vi "Alicat Full Driver Example.vi"() -> ()   [LabVIEW 2015]
doc: "Example program displaying the potential usage of nearly all of the VI's included in the Alicat LabVIEW Driver Library.\n\nThis VI only connects to a single Alicat at a time, and some features may be locked out due to circuit board revision or firmware revision (newer units have additional features available to them).\n\nIf you have any questions regarding the VI's used in this example, please see the Alicat LabVIEW Driver Library Manual (available on the Alicat website and included in the driver library. If you have remaining questions, please contact Alicat at (520) 290-6060 or info@alicat.com."
panel:
  in  "Tare AP Sensor":bool
  in  "Wait message":cluster{"Boolean":bool}
  in  "Read/Write Options":T1 {"Controller Select" items=["No controller"=0, "Volumetric Flow"=36, "Mass Flow"=37, "Absolute Pressure"=34, "Gauge Pressure"=38, "Differential Pressure"=39]}
  out "Batch Units":string="SL"
  in  "Serial Only":T2={"Valve Drive"=FALSE, "Totalizer"=TRUE, "Totalizer Timer"=FALSE, "Totalizer Peak Flow"=FALSE, "Show Abs., Gauge\nand Baro. pressures"=FALSE}
  in  "Data Logging Options":T3={"Absolute Press."=TRUE, "Gauge/Diff. Press."=TRUE, "Barometric Press."=TRUE, "Temperature"=TRUE, "Volumetric"=TRUE, "Mass Flow"=TRUE, "Setpoint"=TRUE, "Valve Drive"=FALSE, "Totalizer"=TRUE, "Tot. Timer [s]"=FALSE, "Tot. Avg. Flow"=FALSE, "Tot. Peak Flow"=FALSE, "Gas Selected"=TRUE, "Log Data"=FALSE}
  out "Measurement Data":T4
  in  "Chart: Manual Scale Adjust":bool
  in  "Chart: AutoScale":bool=TRUE
  out "Chart":T5(graph)
  out "Register value":string
  in  "Reg. to read":u16
  in  "Read Register":bool
  in  "COMPOSER gas mix input":T6={"Mix % 1"=0.0, "Include # 1"=FALSE, "Mix % 2"=0.0, "Include # 2"=FALSE, "Mix % 3"=0.0, "Include # 3"=FALSE, "Mix % 4"=0.0, "Include # 4"=FALSE, "Mix % 5"=0.0, "Include # 5"=FALSE, "COMPOSER gas 1"=0, "COMPOSER gas 2"=0, "COMPOSER gas 3"=0, "COMPOSER gas 4"=0, "COMPOSER gas 5"=0, "Create COMPOSER Mix"=FALSE, "Mix #"=236, "Mix name"="MyMix1", "Completion\ntext"="", "Create COMPOSER Mix 2"=FALSE} {"Mix #" min=236 max=255 step=1; "COMPOSER gas 5" items=["MyMix1"=236]; "COMPOSER gas 4" items=["MyMix1"=236]; "COMPOSER gas 3" items=["MyMix1"=236]; "COMPOSER gas 2" items=["MyMix1"=236]; "COMPOSER gas 1" items=["MyMix1"=236]; "Mix % 1" min=0.0 max=100.0 step=0.01; "Mix % 2" min=0.0 max=100.0 step=0.01; "Mix % 3" min=0.0 max=100.0 step=0.01; "Mix % 4" min=0.0 max=100.0 step=0.01; "Mix % 5" min=0.0 max=100.0 step=0.01}
  in  "Chart: Setpoint":bool=TRUE
  in  "PID Settings":T7 {"P Gain" min=0 max=65535 step=1; "D Gain" min=0 max=65535 step=1; "I Gain" min=0 max=65535 step=1}
  in  "Log Register Values":bool
  out "Meas. per\nsecond [Hz]":dbl caption="Elapsed Time (s)"
  out "Time between\nreadings [ms]":dbl caption="Elapsed Time (s)"
  in  "Chart: Graphing":bool=TRUE
  out "Read-Only Options":T8={"Analog SP"=enum."4-20mA", "Control Invert"=enum."Pressure", "Main PWM"=enum."Volumetric Flow 0-2.5-5V bidir", "Aux PWM"=enum."Fixed 0.00V"}
  in  "Tare Options":T9={"Display"=enum."None", "External"=enum."None", "Auto-Tare Delay [s]"=nan} {"Auto-Tare Delay [s]" min=0.0 max=25.5 step=0.1 format="%.1g"}
  in  "Tare Pressure":bool
  in  "Tare Flow":bool
  in  "Reset Total":bool
  in  "Chart: Mass Flow":bool=TRUE
  in  "Chart: Volumetric":bool=TRUE
  in  "Chart: Temperature":bool=TRUE
  in  "Chart: Pressure":bool=TRUE
  in  "Time between \nreadings [ms]":u32
  out "Totalizer":T10(ring)
  out "Setpoint Units":string="SLPM"
  in  "Serial and Display":T11={"Pressure"=TRUE, "Temperature"=TRUE, "Volumetric"=TRUE, "Mass Flow"=TRUE, "Tot. Avg Flow"=FALSE, "Gas Selected"=TRUE}
  out "(Full Scale)":dbl=nan
  in  "Setpoint":dbl
  in  "Batch Setpoint":dbl format="%.2f"
  in  "Gas Select":u16(ring) items=["MyMix1"=236]
  out "Manufacturer Info":string
  in  "COM Port Settings":T12={"Unit ID"="A", "Baud Rate"=enum."19200", "VISA Sesssion In"="COM1"}
  # "Setpoint and Batching Controls"
  # "Manual Tare"
  # "Data Frame Enables"
  # "Controller Options\nand Analog Signal\nInformation"
  # "(Resetting the Totalizer will reset the batch)"
  # "Graphing Options:"
  # "VI Timing Options"
  # "Register Values"
  # "Populating VI with device information, please wait."
  # "Altering log options will start a new data log"
  # "(The data will be logged to the folder containing the VI)"
  # "Totalizer Timer"
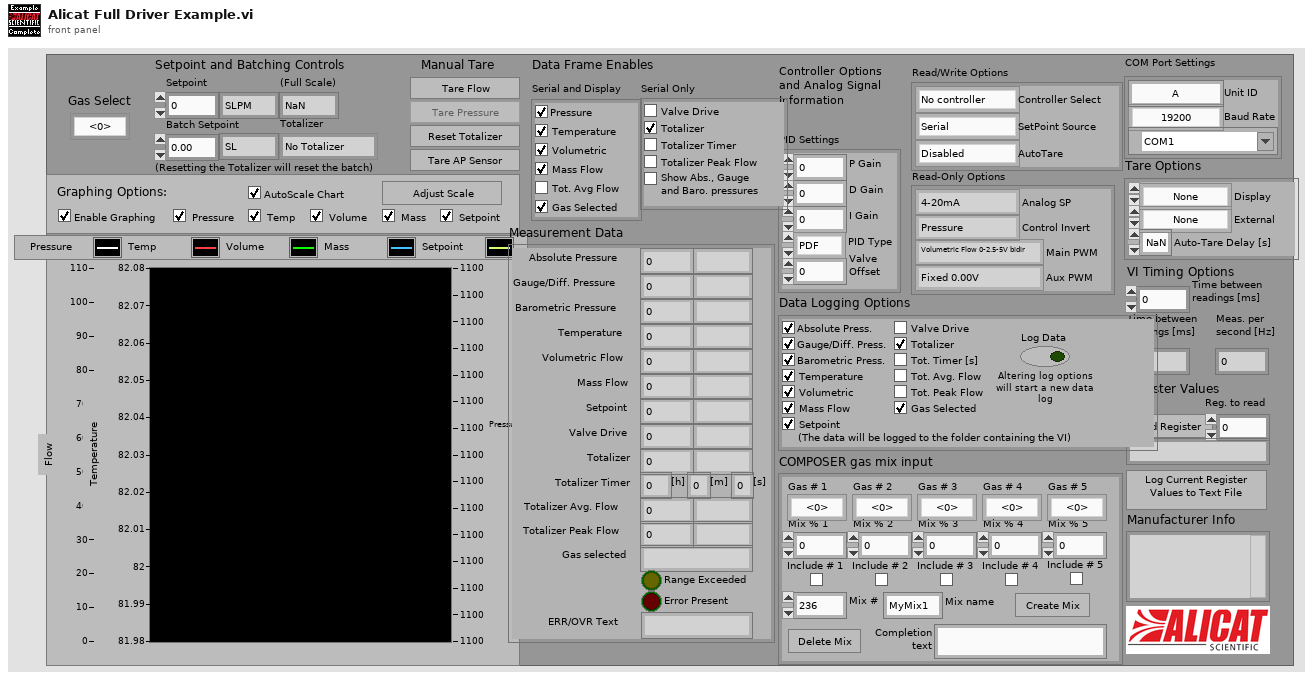
[diagram p1: front panel]
types:
  T1 = cluster{"Controller Select":u16, "SetPoint Source":enum8{"Serial", "Local", "Analog", "Unknown"}, "AutoTare":enum16{"Disabled", "Enabled"}}
  T2 = cluster{"Valve Drive":bool, "Totalizer":bool, "Totalizer Timer":bool, "Totalizer Peak Flow":bool, "Show Abs., Gauge\nand Baro. pressures":bool}
  T3 = cluster{"Absolute Press.":bool, "Gauge/Diff. Press.":bool, "Barometric Press.":bool, "Temperature":bool, "Volumetric":bool, "Mass Flow":bool, "Setpoint":bool, "Valve Drive":bool, "Totalizer":bool, "Tot. Timer [s]":bool, "Tot. Avg. Flow":bool, "Tot. Peak Flow":bool, "Gas Selected":bool, "Log Data":bool}
  T4 = cluster{"Absolute Pressure":dbl, "Gauge/Diff. Pressure":dbl, "Barometric Pressure":dbl, "Temperature":dbl, "Volumetric Flow":dbl, "Mass Flow":dbl, "Setpoint":dbl, "Valve Drive":dbl, "Totalizer":dbl, "[h]":dbl, "[m]":dbl, "[s]":dbl, "Totalizer Avg. Flow":dbl, "Totalizer Peak Flow":dbl, "Gas selected":string, "Range Exceeded":bool, "Error Present":bool, "ERR/OVR Text":string, "Abs. Pressure":string, "Temperature 2":string, "Volume":string, "Mass":string, "Totalizer 2":string, "Valve Drive 2":string, "Gauge/Diff. Press.":string, "Barometric Press.":string, "Setpoint 2":string, "Tot. Avg. Flow":string, "Tot. Peak Flow":string}
  T5 = cluster{"Pressure":dbl, "Temperature":dbl, "Volumetric":dbl, "Mass":dbl, "SetPoint":dbl}
  T6 = cluster{"Mix % 1":dbl, "Include # 1":bool, "Mix % 2":dbl, "Include # 2":bool, "Mix % 3":dbl, "Include # 3":bool, "Mix % 4":dbl, "Include # 4":bool, "Mix % 5":dbl, "Include # 5":bool, "COMPOSER gas 1":u16, "COMPOSER gas 2":u16, "COMPOSER gas 3":u16, "COMPOSER gas 4":u16, "COMPOSER gas 5":u16, "Create COMPOSER Mix":bool, "Mix #":u16, "Mix name":string, "Completion\ntext":string, "Create COMPOSER Mix 2":bool}
  T7 = cluster{"P Gain":i32, "D Gain":i32, "I Gain":i32, "PID Type":enum8{"PDF", "PD2I"}, "Valve \nOffset":i32}
  T8 = cluster{"Analog SP":enum16{"0-5V", "4-20mA"}, "Control Invert":enum16{"Pressure", "Vacuum/BP"}, "Main PWM":enum8{"Fixed 0.00V", "Pressure 0-5V", "Temperature 0-5V", "Volumetric Flow 0-5V", "Mass Flow 0-5V", "Pressure 0-2.5-5V bidir", "Temperature 0-2.5-5V bidir", "Volumetric Flow 0-2.5-5V bidir", "Mass Flow 0-2.5-5V bidir", "Pressure 1-5V", "Temperature 1-5V", "Volumetric Flow 1-5V", "Mass Flow 1-5V", "Reserved(A)", "Reserved(B)", "Fixed 5.12V"}, "Aux PWM":enum8{"Fixed 0.00V", "Pressure 0-5V", "Temperature 0-5V", "Volumetric Flow 0-5V", "Mass Flow 0-5V", "Pressure 0-2.5-5V bidir", "Temperature 0-2.5-5V bidir", "Volumetric Flow 0-2.5-5V bidir", "Mass Flow 0-2.5-5V bidir", "Pressure 1-5V", "Temperature 1-5V", "Volumetric Flow 1-5V", "Mass Flow 1-5V", "Reserved(A)", "Reserved(B)", "Fixed 5.12V"}}
  T9 = cluster{"Display":enum16{"None", "Pressure", "Volumetric"}, "External":enum16{"None", "Pressure", "Volumetric", "Totalizer"}, "Auto-Tare Delay [s]":dbl}
  T10 = enum8{"No Totalizer", "Mass Flow", "Volumetric Flow"}
  T11 = cluster{"Pressure":bool, "Temperature":bool, "Volumetric":bool, "Mass Flow":bool, "Tot. Avg Flow":bool, "Gas Selected":bool}
  T12 = cluster{"Unit ID":string, "Baud Rate":enum8{"2400", "9600", "19200", "38400", "57600", "115200", "Unknown"}, "VISA Sesssion In":refnum<visa-resource-name>}
  T13 = cluster{"Absolute Pressure":bool, "Gauge/Diff. Pressure":bool, "Barometric Pressure":bool, "Temperature":bool, "Volumetric":bool, "Mass":bool, "Setpoint":bool, "Valve Drive":bool, "Totalizer":bool, "Totalizer Timer":bool, "Totalizer Average Flow":bool, "Totalizer Peak Flow":bool, "Gas Selected":bool, "Tot. Timer Format":u16}
  T14 = cluster{"Controller Full Scale":dbl, "Controller Select":u16, "Control Range":enum16{"Normal", "Inverted", "Bidirectional", "Unknown"}}
  T15 = cluster{"Absolute Pressure":dbl, "Gauge/Diff. Pressure":dbl, "Barometric Pressure":dbl, "Temperature":dbl, "Volumetric Flow":dbl, "Mass Flow":dbl, "Setpoint":dbl, "Valve Drive":dbl, "Totalizer":dbl, "[h]":dbl, "[m]":dbl, "[s]":dbl, "Totalizer Average Flow":dbl, "Totalizer Peak Flow":dbl, "Gas selected":string, "Range Exceeded":bool, "Error Present":bool, "ERR/OVR Text":string, "Abs. Pressure":string, "Temperature 2":string, "Volume":string, "Mass":string, "Totalizer 2":string, "Valve Drive 2":string, "Gauge/Diff. Press.":string, "Barometric Press.":string, "Setpoint 2":string, "Tot. Avg. Flow":string, "Tot. Peak Flow":string}
  T16 = cluster{"Abs. Pressure":string, "Gauge/Diff. Press.":string, "Barometric Press.":string, "Temperature":string, "Volume":string, "Mass":string, "Setpoint":string, "Valve Drive":string, "Totalizer":string, "Tot. Timer":string, "Tot. Avg. Flow":string, "Tot. Peak Flow":string}
  T17 = cluster{"Pressure":bool, "Temperature":bool, "Volumetric":bool, "Mass Flow":bool, "Setpoint":bool, "Chart: AutoScale":bool}
  T18 = cluster{"Enabled":enum8{"Enabled", "Disabled", "Disabled and Grayed Out"}, "Disabled and Grayed Out":enum8{"Enabled", "Disabled", "Disabled and Grayed Out"}}
  T19 = cluster{"Absolute Pressure":dbl, "Gauge/Diff. Pressure":dbl, "Barometric Pressure":dbl, "Temperature":dbl, "Volumetric":dbl, "Mass Flow":dbl, "Setpoint":dbl, "Valve Drive":dbl, "Totalizer":dbl, "[hr]":dbl, "[min]":dbl, "[sec]":dbl, "Totalizer Average Flow":dbl, "Totalizer Peak Flow":dbl, "Gas selected":string}
  T20 = cluster{"Pressure(s)":bool, "Temperature":bool, "Volumetric":bool, "Mass":bool, "Totalizer Average Flow":bool, "Gas Selected":bool}
  T21 = enum16{"open", "replace", "create", "open or create", "replace or create", "replace or create with confirmation"}
  T22 = cluster{"P Gain":i32, "D Gain":i32, "I Gain":i32}
  T23 = cluster{"PID Type":enum8{"PDF", "PD2I"}, "Valve Offset":i32}
  T24 = cluster{"Gas # 1":u16, "Mix % 1":dbl, "Include # 1":bool, "Gas # 2":u16, "Mix % 2":dbl, "Include # 2":bool, "Gas # 3":u16, "Mix % 3":dbl, "Include # 3":bool, "Gas # 4":u16, "Mix % 4":dbl, "Include # 4":bool, "Gas # 5":u16, "Mix % 5":dbl, "Include # 5":bool}
  T25 = cluster{"Pressure":bool, "Temperature":bool, "Volumetric":bool, "Mass":bool, "Totalizer Average Flow":bool, "Gas Selected":bool}
  T26 = enum8{"Enabled", "Disabled", "Disabled and Grayed Out"}
  T27 = enum16{"None", "Pressure", "Volumetric", "Totalizer"}
  T28 = cluster{"Valve Amount":enum8{"Single Valve", "Dual Valve"}, "PID Type":enum8{"PDF", "PD2I"}, "Valve Offset":i32, "P Gain":i32, "D Gain":i32, "I Gain":i32}
  T29 = cluster{"Absolute Pressure":dbl, "Gauge/Diff. Pressure":dbl, "Volumetric Flow":dbl, "Mass Flow":dbl}
  T30 = cluster{"Absolute Pressure":dbl, "Gauge/Diff. Pressure":dbl, "Barometric Pressure":dbl, "Temperature":dbl, "Volumetric Flow":dbl, "Mass Flow":dbl, "Setpoint":dbl, "Valve Drive":dbl, "Totalizer":dbl, "[hr]":dbl, "[min]":dbl, "[sec]":dbl, "Totalizer Average Flow":dbl, "Totalizer Peak Flow":dbl, "Gas selected":string}
  T31 = enum8{"2400", "9600", "19200", "38400", "57600", "115200", "Unknown"}
  T32 = cluster{"Pressure":bool, "Temperature":bool, "Volumetric":bool, bool, bool, "Gas Selected":bool}
  T33 = enum16{"Left Button", "Center Button", "Right Button", "Window Close"}
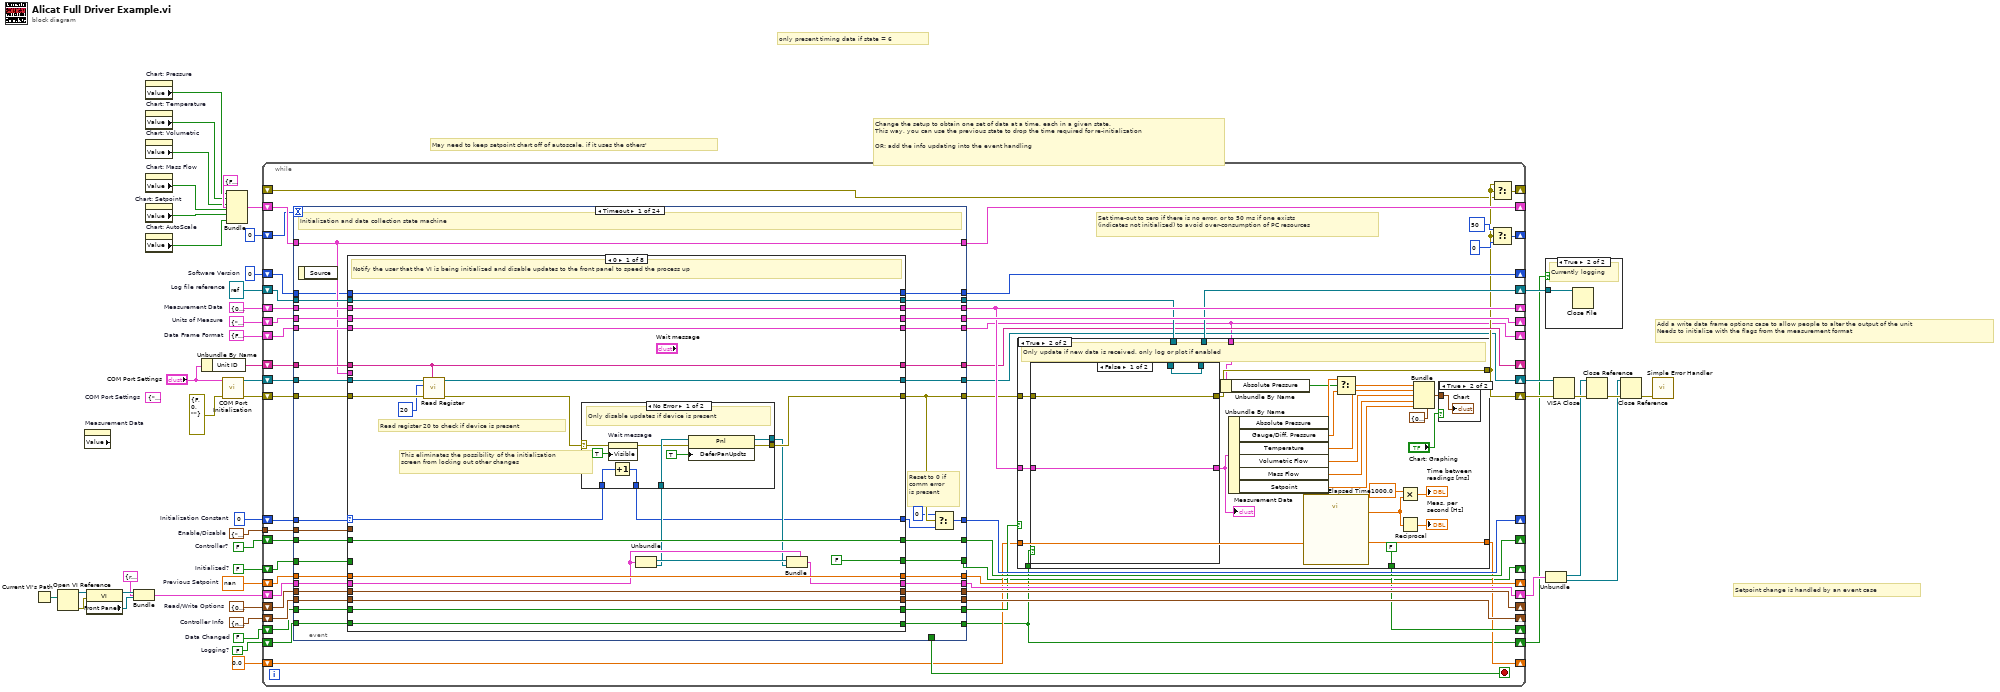
[diagram p0: block diagram]
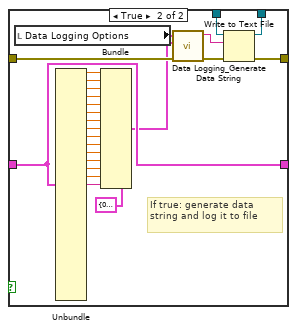
[diagram p5: hidden frame]
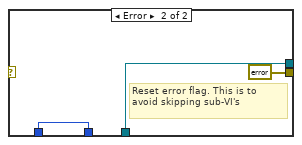
[diagram p6: hidden frame]
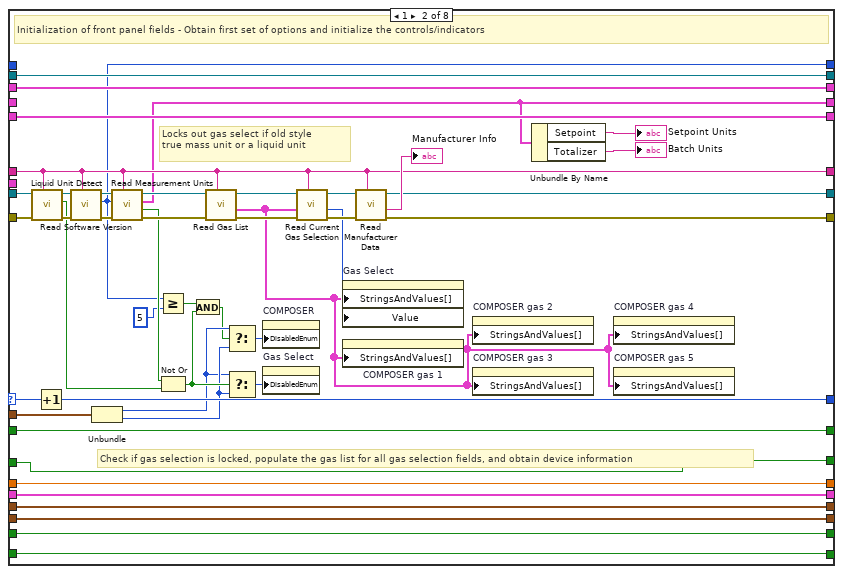
[diagram p7: hidden frame]
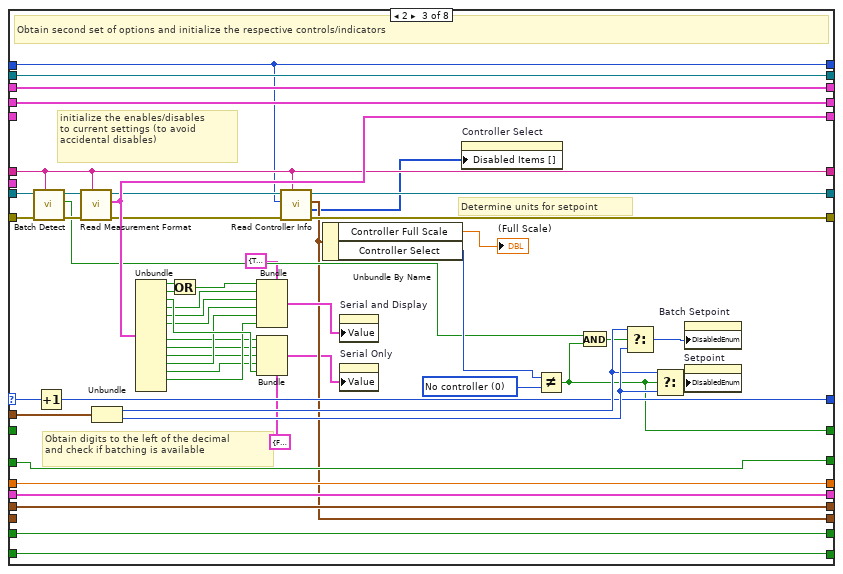
[diagram p8: hidden frame]
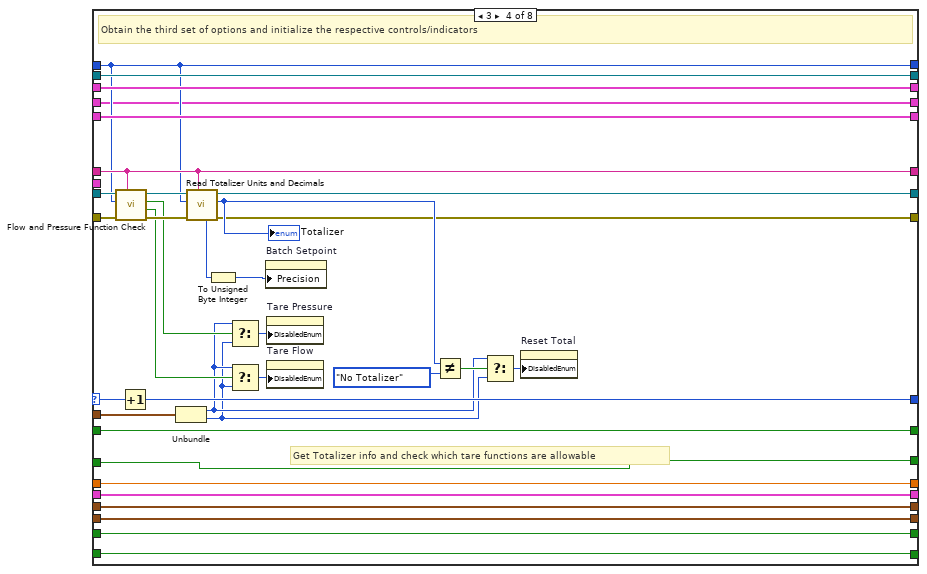
[diagram p9: hidden frame]
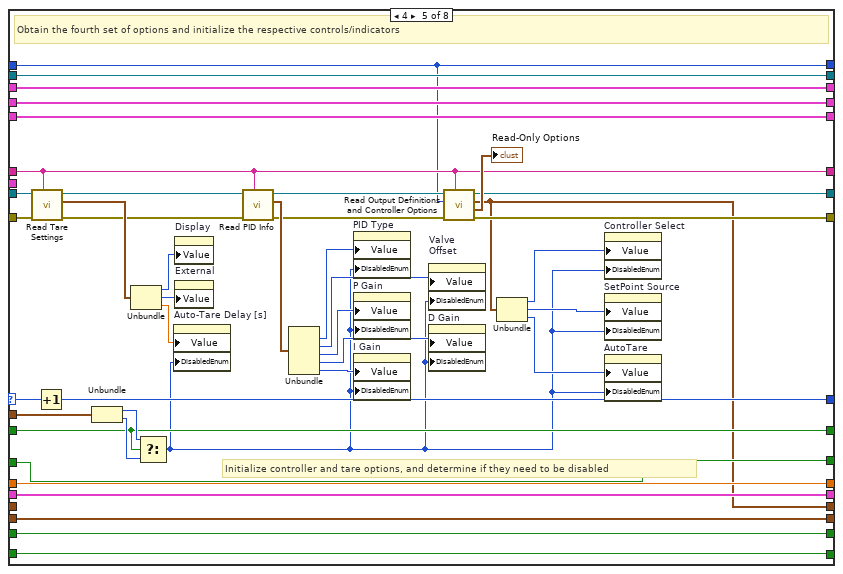
[diagram p10: hidden frame]
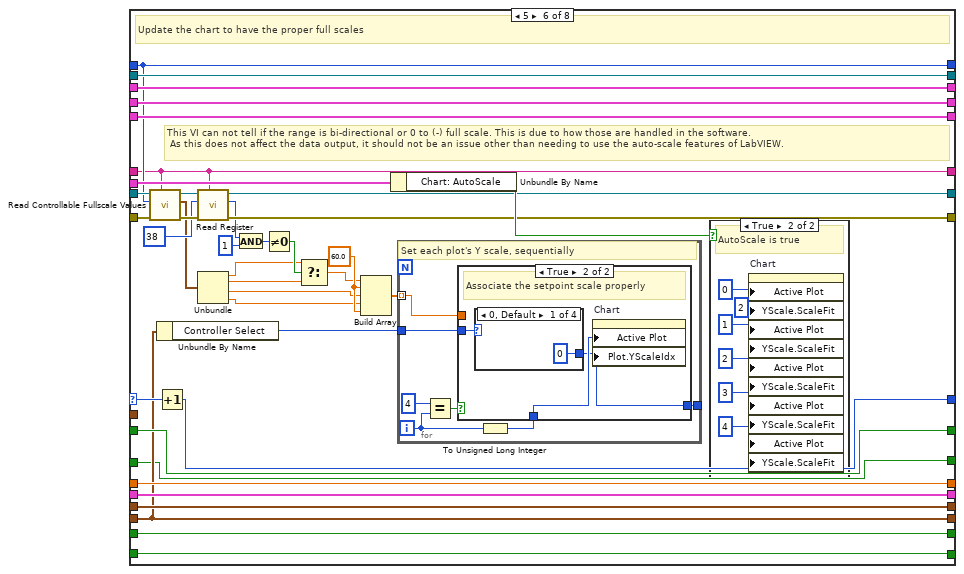
[diagram p11: hidden frame]
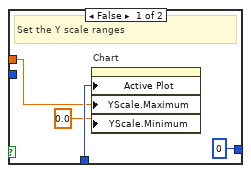
[diagram p13: hidden frame]
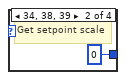
[diagram p14: hidden frame]
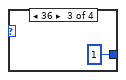
[diagram p15: hidden frame]
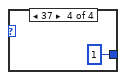
[diagram p16: hidden frame]
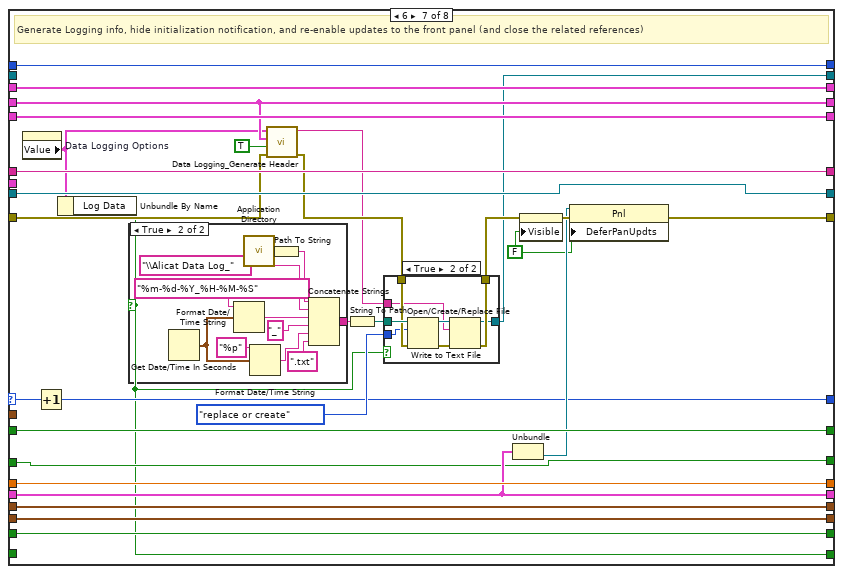
[diagram p17: hidden frame]
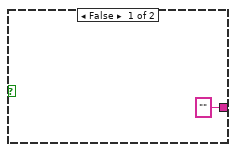
[diagram p18: hidden frame]
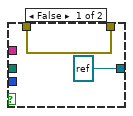
[diagram p19: hidden frame]
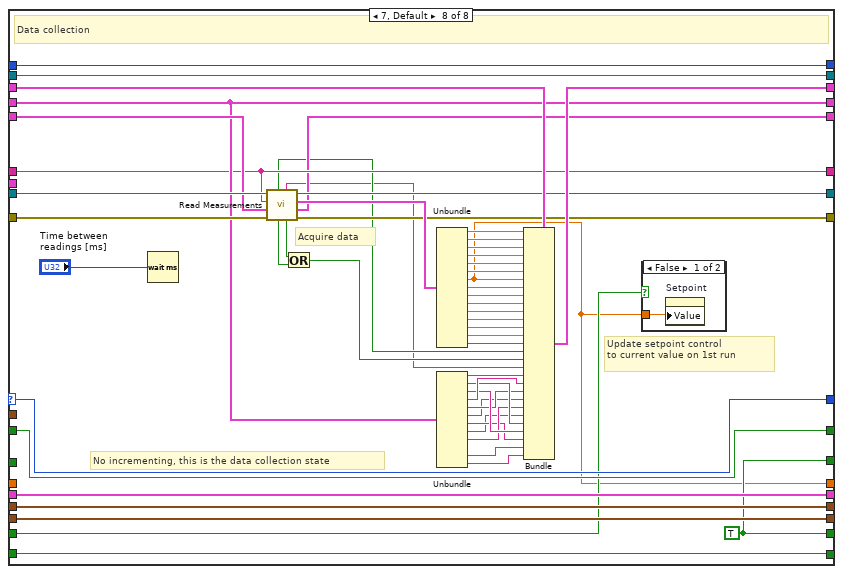
[diagram p20: hidden frame]
diagram:
  w1 = T13 {"Absolute Pressure"=FALSE, "Gauge/Diff. Pressure"=FALSE, "Barometric Pressure"=FALSE, "Temperature"=FALSE, "Volumetric"=FALSE, "Mass"=FALSE, "Setpoint"=FALSE, "Valve Drive"=FALSE, "Totalizer"=FALSE, "Totalizer Timer"=FALSE, "Totalizer Average Flow"=FALSE, "Totalizer Peak Flow"=FALSE, "Gas Selected"=FALSE, "Tot. Timer Format"=0}  # Data Frame Format
  w2 = T1 {"Controller Select"=0, "SetPoint Source"=enum."Serial", "AutoTare"=enum."Disabled"}  # Read/Write Options
  w3 = T14 {"Controller Full Scale"=nan, "Controller Select"=0, "Control Range"=enum."Normal"}  # Controller Info
  (unwired) T12 {"Unit ID"="A", "Baud Rate"=enum."19200", "VISA Sesssion In"="COM1"}  # COM Port Settings
  w4 = T15 {"Absolute Pressure"=0.0, "Gauge/Diff. Pressure"=0.0, "Barometric Pressure"=0.0, "Temperature"=0.0, "Volumetric Flow"=0.0, "Mass Flow"=0.0, "Setpoint"=0.0, "Valve Drive"=0.0, "Totalizer"=0.0, "[h]"=0.0, "[m]"=0.0, "[s]"=0.0, "Totalizer Average Flow"=0.0, "Totalizer Peak Flow"=0.0, "Gas selected"="", "Range Exceeded"=FALSE, "Error Present"=FALSE, "ERR/OVR Text"="", "Abs. Pressure"="", "Temperature 2"="", "Volume"="", "Mass"="", "Totalizer 2"="", "Valve Drive 2"="", "Gauge/Diff. Press."="", "Barometric Press."="", "Setpoint 2"="", "Tot. Avg. Flow"="", "Tot. Peak Flow"=""}  # Measurement Data
  w5 = T16 {"Abs. Pressure"="", "Gauge/Diff. Press."="", "Barometric Press."="", "Temperature"="", "Volume"="", "Mass"="", "Setpoint"="", "Valve Drive"="", "Totalizer"="", "Tot. Timer"="", "Tot. Avg. Flow"="", "Tot. Peak Flow"=""}  # Units of Measure
  w6 = u8 0  # Software Version
  w8 = FALSE  # Logging?
  w9 = FALSE  # Initialized?
  w25 = FALSE  # Data Changed
  w27 = refnum<file> refnum  # Log file reference
  w37 = nan  # Previous Setpoint
  w38 = FALSE  # Controller?
  w39 = T18 {"Enabled"=enum."Enabled", "Disabled and Grayed Out"=enum."Disabled and Grayed Out"}  # Enable/Disable
  w40 = 0  # Initialization Constant
  # "May need to keep setpoint chart off of autoscale, if it uses the others'"
  # "only present timing data if state = 6"
  # "Change the setup to obtain one set of data at a time, each in a given state.\nThis way, you can use the previous state to drop the time required for re-initialization\n\nOR: add the info updating into the event handling"
  # "Setpoint change is handled by an event case"
  # "Add a write data frame options case to allow people to alter the output of the unit\nNeeds to initialize with the flags from the measurement format"
  n1 = Current VI's Path() -> (path=w34:path)
  n2 = Open VI Reference(vi path=w34) -> (vi reference=w32:refnum<vi>, error out=w33:errorcluster)  [unwired: 2 in, 3 out]
  n3 = property on="Measurement Data" class="Clust (strict)" props=["Value"]() -> ()  [unwired: 2 in, 3 out]
  n4 = property class="VI"(reference=w32, error in=w33) -> (reference out=w30:refnum<vi>, "Front Panel"=w31:refnum<vi>)  [unwired: 1 out]
  n5 = Bundle(cluster=cluster{refnum<vi>, "Panel":refnum<vi>} {refnum, "Panel"=refnum}, w30, "Panel"=w31) -> (w29:cluster{refnum<vi>, "Panel":refnum<vi>})
  n6 = property on="Chart: Pressure" class="Bool (strict)"() -> ("Value"=w19:bool)  [unwired: 2 in, 2 out]
  n7 = property on="Chart: Temperature" class="Bool (strict)"() -> ("Value"=w20:bool)  [unwired: 2 in, 2 out]
  n8 = property on="Chart: Volumetric" class="Bool (strict)"() -> ("Value"=w21:bool)  [unwired: 2 in, 2 out]
  n9 = property on="Chart: Mass Flow" class="Bool (strict)"() -> ("Value"=w22:bool)  [unwired: 2 in, 2 out]
  n10 = property on="Chart: Setpoint" class="Bool (strict)"() -> ("Value"=w23:bool)  [unwired: 2 in, 2 out]
  n11 = property on="Chart: AutoScale" class="Bool (strict)"() -> ("Value"=w17:bool)  [unwired: 2 in, 2 out]
  n12 = Unbundle By Name("COM Port Settings") -> ("Unit ID"=w41:string)
  n13 = call "COM Port Initialization.vi"("error in (no error)"=errorcluster {"status"=FALSE, "code"=0, "source"=""}, "Communication Settings"="COM Port Settings") -> ("error out"=w44:errorcluster, "VISA Session Out"=w46:refnum<visa-resource-name>)  [unwired: 8 in]
  n14 = Bundle(cluster=T17 {"Pressure"=FALSE, "Temperature"=FALSE, "Volumetric"=FALSE, "Mass Flow"=FALSE, "Setpoint"=FALSE, "Chart: AutoScale"=TRUE} ("Graphing enables"), "Pressure"=w19, "Temperature"=w20, "Volumetric"=w21, "Mass Flow"=w22, "Setpoint"=w23, "Chart: AutoScale"=w17) -> (w35:T17)
  n15 = while {
    shift-right: [w91] -> _
    shift-left: w40 -> [w92]
    shift-right: [w73] -> _
    shift-left: w4 -> [w90]
    shift-right: [w88] -> _
    shift-left: w5 -> [w89]
    tunnel: w39 -> [w87]
    shift-right: [w47] -> _
    shift-left: w1 -> [w86]
    shift-right: [w48] -> w45
    shift-left: w46 -> [w95]
    shift-right: [w51] -> w43
    shift-left: w44 -> [w94]
    shift-right: [w52] -> _
    shift-left: w41 -> [w93]
    shift-right: [w85] -> _
    shift-left: w38 -> [w84]
    shift-right: [w83] -> _
    shift-left: w37 -> [w82]
    shift-right: [w63] -> _
    shift-left: w35 -> [w64]
    shift-right: [w80] -> w12
    shift-left: w29 -> [w81]
    shift-right: [w77] -> _
    shift-left: w2 -> [w78]
    shift-right: [w75] -> _
    shift-left: w3 -> [w76]
    shift-right: [w67] -> w26
    shift-left: w27 -> [w74]
    shift-right: [w71] -> _
    shift-left: w25 -> [w72]
    shift-right: [w66] -> _
    shift-left: 0.0 ("Get Start Time (s)") -> [w65]
    shift-right: [w59] -> _
    shift-left: 0 -> [w60]
    shift-right: [w57] -> _
    shift-left: w9 -> [w58]
    shift-right: [w55] -> w7
    shift-left: w8 -> [w56]
    shift-right: [w54] -> _
    shift-left: w6 -> [w53]
    shift-right: [w50] -> _
    shift-left: _ -> [w49]
    stop <- w79 stop-if-true
    # "Set time-out to zero if there is no error, or to 50 ms if one exists\n(indicates not initialized) to avoid over-consumption of PC resources"
    n16 = event shown="[0] Timeout" {
      selector: _ -> [_ _ _ _ _ _ _ _ _ _ _ _ _ _ _ _ _ _ _ _ _ _ _ _]
      dyn-events: _ -> [_ _ _ _ _ _ _ _ _ _ _ _ _ _ _ _ _ _ _ _ _ _ _ _]
      timeout: w60 -> [_ _ _ _ _ _ _ _ _ _ _ _ _ _ _ _ _ _ _ _ _ _ _ _]
      tunnel: [w188 w586 w608 w626 w655 w671 w692 w713 w734 w757 w779 w813 w837 w870 w885 w943 w972 w998 w1016 w1108 w1138 w1158 w1207 w1260] -> w48
      tunnel: w95 -> [w192 w586 w604 w627 w655 w670 w691 w712 w733 w758 w780 w802 w843 w863 w915 w944 w973 w988 w1065 w1112 w1138 w1158 w1207 w1260]
      tunnel: w94 -> [w191 w585 w605 w629 w654 w673 w694 w715 w736 w755 w777 w822 w844 w862 w914 w941 w971 w987 w1064 w1111 w1139 w1159 w1197 w1243]
      tunnel: [w171 w585 w609 w628 w654 w672 w693 w714 w735 w756 w778 w812 w836 w869 w880 w942 w959 w996 w1055 w1088 w1139 w1159 w1188 w1257] -> w69
      tunnel: w93 -> [w190 w587 w614 w635 _ w669 w690 w711 w732 w753 w776 w797 w835 w868 w884 w940 w970 w983 w1015 w1105 w1137 w1157 w1206 w1259]
      tunnel: w92 -> [w189 w584 _ _ _ w674 w695 w716 w737 w759 w781 w814 w845 w871 w916 w945 w974 w999 w1066 w1113 w1142 w1162 w1210 w1263]
      tunnel: [w172 w584 0 ("Initialization Constant") 0 ("Initialization Constant") 0 ("t") w675 w696 w717 w738 w760 w782 w815 w846 w872 w917 w946 w975 w1000 w1067 w1114 w1143 w1163 w1211 w1264] -> w91
      tunnel: w90 -> [w187 w590 w616 w637 w661 w682 w703 w724 w745 w767 w789 w821 w853 w879 w924 w953 w982 w1007 w1014 w1120 w1149 w1169 w1217 w1269]
      tunnel: [w178 w590 w616 w637 w661 w682 w703 w724 w745 w767 w789 w821 w853 w879 w924 w953 w982 w1007 w1013 w1120 w1149 w1169 w1217 w1269] -> w73
      tunnel: w89 -> [w186 w589 w615 w636 w660 w681 w702 w723 w744 w766 w788 w820 w852 w878 w923 w952 w981 w1006 w1022 w1119 w1148 w1168 w1216 w1251]
      tunnel: [w185 w589 w615 w636 w660 w681 w702 w723 w744 w766 w788 w820 w852 w878 w923 w952 w981 w1006 w1022 w1119 w1148 w1168 w1216 w1251] -> w88
      tunnel: w87 -> [w184 _ _ _ _ _ _ _ _ _ _ _ _ _ _ _ _ _ _ _ _ _ _ _]
      tunnel: w86 -> [w183 w588 w613 w634 w659 w680 w701 w722 w743 w765 w787 w819 w851 w877 w922 w951 w980 w1005 w1011 _ w1136 w1156 w1183 w1248]
      tunnel: [w182 w587 w614 w635 w652 w669 w690 w711 w732 w753 w776 w797 w835 w868 w884 w940 w970 w983 w1015 w1105 w1137 w1157 w1206 w1259] -> w52
      tunnel: [w181 w588 w613 w634 w659 w680 w701 w722 w743 w765 w787 w819 w851 w877 w922 w951 w980 w1005 w1010 w1103 w1136 w1156 w1183 w1248] -> w47
      tunnel: [w180 w583 w612 w633 w658 w679 w700 w721 w742 w764 w786 w798 w850 w876 w921 w950 w979 w1004 w1070 w1118 w1147 w1167 w1215 w1268] -> w85
      tunnel: w84 -> [w179 w583 w612 w633 w658 w679 w700 w721 w742 w764 w786 w798 w850 w876 w921 w950 w979 w1004 w1070 w1118 w1147 w1167 w1215 w1268]
      tunnel: w82 -> [w177 w582 w611 w632 w657 w678 w699 w720 w741 w763 w785 w818 w849 w875 w920 w949 w978 w1003 w1062 w1117 w1146 w1166 w1214 w1267]
      tunnel: [w176 w582 w611 w632 w657 w678 w699 w720 w741 w763 w785 w818 w849 w875 w920 w949 w978 w1003 w1009 w1117 w1146 w1166 w1214 w1267] -> w83
      tunnel: w81 -> [w175 w581 w610 w631 w656 w677 w698 w719 w740 w762 w784 w817 w848 w874 w919 w948 w977 w1002 w1069 w1116 w1145 w1165 w1213 w1266]
      tunnel: [w174 w581 w610 w631 w656 w677 w698 w719 w740 w762 w784 w817 w848 w874 w919 w948 w977 w1002 w1069 w1116 w1145 w1165 w1213 w1266] -> w80
      tunnel: [_ w591 _ _ _ _ _ _ _ _ _ _ _ _ _ _ _ _ _ _ _ _ _ _] -> w79
      tunnel: w78 -> [w169 w580 w603 w623 w651 w668 w689 w710 w731 w752 w774 w811 w834 w860 w892 w931 w969 w997 w1063 w1110 w1141 w1161 w1209 w1262]
      tunnel: [w168 w580 w603 w623 w651 w668 w689 w710 w731 w752 w774 w808 w834 w860 w892 w931 w969 w997 w1063 w1110 w1141 w1161 w1209 w1262] -> w77
      tunnel: w76 -> [w167 w579 w602 w622 w650 w667 w688 w709 w730 w751 w773 w807 w833 w859 w891 w930 w968 w994 w1057 w1109 w1140 w1160 w1208 w1261]
      tunnel: [w166 w579 w602 w622 w650 w667 w688 w709 w730 w751 w773 w807 w833 w859 w891 w930 w968 w994 w1056 w1109 w1140 w1160 w1208 w1261] -> w75
      tunnel: [w165 w578 w601 w621 w649 w666 w687 w708 w729 w750 w772 w806 w832 w858 w890 w929 w958 w993 w1054 w1102 w1135 w1155 w1205 w1252] -> w68
      tunnel: w74 -> [w164 w578 w601 w621 w649 w666 w687 w708 w729 w750 w772 w806 w832 w858 w890 w929 w958 w993 w1054 w1102 w1135 w1155 w1205 w1244]
      tunnel: w72 -> [w163 _ _ _ _ _ _ _ _ _ _ _ _ _ _ _ _ _ _ _ _ _ _ _]
      tunnel: [w162 _ _ _ _ _ _ _ _ _ _ _ _ _ _ _ _ _ TRUE ("Data Changed") _ _ _ _ _] -> w70
      tunnel: w64 -> [w161 w577 w600 w620 w648 w665 w686 w707 w728 w749 w771 w796 w831 w857 w889 w928 w957 w992 w1051 w1100 w1134 w1154 w1204 w1247]
      tunnel: [w161 w577 w600 w620 w648 w665 w686 w707 w728 w749 w771 w796 w831 w857 w889 w928 w957 w992 w1051 w1100 w1134 w1154 w1204 w1247] -> w63
      tunnel: w58 -> [w160 w576 w599 w619 w647 w664 w685 w706 w727 w748 w770 w795 w830 w856 w888 w927 w956 w991 w1050 w1099 w1123 w1152 w1185 w1246]
      tunnel: [w159 w576 w599 w619 w647 w664 w685 w706 w727 w748 w770 w795 w830 w856 w888 w927 w956 w991 w1050 w1099 w1123 w1152 w1185 w1246] -> w57
      tunnel: w56 -> [w158 w575 w598 w618 w646 w663 w684 w705 w726 w747 w769 w794 w829 w855 w883 w926 w955 w990 w1049 w1090 w1122 w1151 w1184 w1241]
      tunnel: [w157 w575 w598 w618 w646 w663 w684 w705 w726 w747 w769 w794 w829 w855 w883 w926 w955 w990 w1049 w1090 w1122 w1151 w1184 w1245] -> w55
      tunnel: [w156 w574 w597 w617 w645 w662 w683 w704 w725 w746 w768 w792 w827 w854 w882 w925 w954 w989 w1008 w1087 w1121 w1150 w1182 w1239] -> w54
      tunnel: w53 -> [w155 w574 w597 w617 w645 w662 w683 w704 w725 w746 w768 w792 w827 w854 w882 w925 w954 w989 w1008 w1087 w1121 w1150 w1182 w1239]
      event Timeout {
        # "Reset to 0 if\ncomm error\nis present"
        # "Initialization and data collection state machine"
        n17 = event-data() -> ()  [unwired: 1 in, 1 out]
        n18 = case shown="0" w189 {
          selector: w189 -> [w196 w276 w328 w343 w403 w435 w473 w547]
          tunnel: w192 -> [w206 w265 w297 w362 w382 w424 w495 w558]
          tunnel: w191 -> [w207 w264 w296 w363 w383 w423 w486 w557]
          tunnel: w190 -> [w204 w251 w316 w341 w391 w416 w494 w552]
          tunnel: [w195 w275 w311 w342 w401 w434 w474 w547] -> w173
          tunnel: [w205 w263 w317 w345 w378 w421 w495 w551] -> w188
          tunnel: [w213 w262 w318 w346 w379 w420 w475 w550] -> w171
          tunnel: w187 -> [w216 w261 w323 w348 w400 w441 w492 w571]
          tunnel: [w216 w261 w323 w348 w400 w441 w492 w570] -> w178
          tunnel: [w217 w233 w300 w329 w399 w442 w485 w555] -> w185
          tunnel: w186 -> [w217 _ w300 w329 w399 w442 w485 w555]
          tunnel: w184 -> [_ w260 w322 w355 w402 _ _ _]
          tunnel: [w218 w259 w321 w347 w398 w443 w493 w537] -> w181
          tunnel: w183 -> [w218 w259 _ w347 w398 w443 w493 w556]
          tunnel: [w204 w251 w316 w341 w391 w416 w494 w552] -> w182
          tunnel: [w215 w258 w307 w344 w384 w439 w496 w549] -> w180
          tunnel: w179 -> [w215 w258 _ w344 w384 w439 w496 w549]
          tunnel: w177 -> [w214 w257 w310 w340 w404 w438 w497 _]
          tunnel: [w214 w257 w310 w340 w404 w438 w497 w536] -> w176
          tunnel: w175 -> [w211 w256 w309 w339 w375 w437 w491 w545]
          tunnel: [w208 w256 w309 w339 w375 w437 w491 w545] -> w174
          tunnel: w169 -> [w201 w240 w305 w336 _ w436 w488 w543]
          tunnel: [w201 w240 w305 w336 w369 w436 w488 w543] -> w168
          tunnel: w167 -> [w200 w239 _ w335 w374 w433 w487 w544]
          tunnel: [w200 w239 w298 w335 w374 w433 w487 w544] -> w166
          tunnel: [w199 w238 w304 w334 w373 w440 w478 w542] -> w165
          tunnel: w164 -> [w199 w238 w304 w334 w373 w440 _ w542]
          tunnel: w163 -> [w198 w237 w303 w333 w372 w431 w476 w540]
          tunnel: [w198 w237 w303 w333 w372 w431 w476 w541] -> w162
          tunnel: w161 -> [_ _ _ _ _ w428 _ _]
          tunnel: w160 -> [_ w236 w302 w332 w371 w426 w472 _]
          tunnel: [FALSE ("Data Changed") w236 w302 w332 w371 w426 w472 w541] -> w159
          tunnel: w158 -> [w194 w235 w301 w331 w370 w425 _ w539]
          tunnel: [w194 w235 w301 w331 w370 w425 w471 w539] -> w157
          tunnel: [w193 w234 w299 w330 w368 w422 w469 w538] -> w156
          tunnel: w155 -> [w193 _ w299 w330 w368 w422 w469 w538]
          frame 0 {
            # "This eliminates the possibility of the initialization\nscreen from locking out other changes"
            # "Read register 20 to check if device is present"
            # "Notify the user that the VI is being initialized and disable updates to the front panel to speed the process up"
            n19 = call "Read Register.vi"("Unit ID (A)"=w204, "error in"=w207, "Register address"=u16 20, "VISA Session In"=w206) -> ("error out"=w203:errorcluster, "VISA Session Out"=w205:refnum<visa-resource-name>)  [unwired: 5 in, 1 out]
            n20 = Unbundle(w211) -> (w212:refnum<vi>, "Panel"=w209:refnum<vi>)
            n21 = case shown="No Error" w203 {
              selector: w203 -> [w221 _]
              tunnel: [w226 errorcluster {"status"=FALSE, "code"=0, "source"=""} ("error out")] -> w213
              tunnel: [w225 w230] -> w210
              tunnel: w209 -> [w224 w230]
              tunnel: w196 -> [w220 w228]
              tunnel: [w219 w228] -> w195
              frame No Error {
                # "Only disable updates if device is present"
                n22 = property on="Wait message" class="Clust (strict)"(error in=w221, "Visible"=TRUE) -> (error out=w222:errorcluster)  [unwired: 1 in, 1 out]
                n23 = Increment(x=w220) -> (x+1=w219:i32)
                n24 = property class="Pnl"(reference=w224, error in=w222, "DeferPanUpdts"=TRUE ("Defer Panel Updates")) -> (reference out=w225:refnum<vi>, error out=w226:errorcluster)
              }
              frame Error {
                # "Reset error flag. This is to\navoid skipping sub-VI's"
              }
            }
            n25 = Bundle(cluster=w211, w212, "Panel"=w210) -> (w208:cluster{refnum<vi>, "Panel":refnum<vi>})
          }
          frame 1 {
            # "Check if gas selection is locked, populate the gas list for all gas selection fields, and obtain device information"
            # "Locks out gas select if old style\ntrue mass unit or a liquid unit"
            # "Initialization of front panel fields - Obtain first set of options and initialize the controls/indicators"
            n26 = call "Liquid Unit Detect.vi"("Unit ID (A)"=w251, "error in"=w264, "VISA Session In"=w265) -> ("error out"=w269:errorcluster, "Liquid Device"=w267:bool, "VISA Session Out"=w270:refnum<visa-resource-name>)  [unwired: 6 in]
            n27 = Increment(x=w276) -> (x+1=w275:i32)
            n28 = call "Read Software Version.vi"("Unit ID (A)"=w251, "error in"=w269, "VISA Session In"=w270) -> ("error out"=w273:errorcluster, "Software Version"=w234:u8, "VISA Session Out"=w274:refnum<visa-resource-name>)  [unwired: 6 in]
            n29 = Unbundle(w260) -> ("Enabled"=w242:T26, "Disabled and Grayed Out"=w243:T26)
            n30 = call "Read Measurement Units.vi"("Unit ID (A)"=w251, "error in"=w273, "Software Rev"=w234, "VISA Session In"=w274) -> ("error out"=w272:errorcluster, "Lock Gas Select"=w268:bool, "Measurement Units"=w233:T16, "VISA Session Out"=w271:refnum<visa-resource-name>)  [unwired: 4 in]
            n31 = Greater Or Equal?(x=w234, y=u8 5) -> (x >= y?=w247:bool)
            n32 = Not Or(1:w267, 2:w268) -> (0:w246:bool)
            n33 = And(x=w247, y=w246) -> (x .and. y?=w241:bool)
            n34 = call "Read Gas List.vi"("Unit ID (A)"=w251, "error in"=w272, "VISA Session In"=w271) -> ("error out"=w255:errorcluster, "Gas Selection: Strings and Values"=w249:cluster{"Gas Name":string, "Gas number":u16}[], "VISA Session Out"=w252:refnum<visa-resource-name>)  [unwired: 5 in, 1 out]
            n35 = Select(t=w242, s=w241, f=w243) -> (s? t:f=w244:T26)
            n36 = Select(t=w242, s=w246, f=w243) -> (s? t:f=w245:T26)
            n37 = property on="COMPOSER" class="Clust"("DisabledEnum"=w244) -> ()  [unwired: 2 in, 2 out]
            n38 = property on="Gas Select" class="Ring (strict)"("DisabledEnum"=w245) -> ()  [unwired: 2 in, 2 out]
            n39 = call "Read Current Gas Selection.vi"("Unit ID (A)"=w251, "error in"=w255, "Gas Selection: Strings and Values"=w249, "VISA Session In"=w252) -> ("error out"=w254:errorcluster, "Current Gas Selection (number)"=w250:u16, "VISA Session Out"=w253:refnum<visa-resource-name>)  [unwired: 4 in, 1 out]
            n40 = property on="Gas Select" class="Ring (strict)"("StringsAndValues[]"=w249, "Value"=w250) -> ()  [unwired: 2 in, 2 out]
            n41 = property on="COMPOSER gas 1" class="Ring (strict)"("StringsAndValues[]"=w249) -> ()  [unwired: 2 in, 2 out]
            n42 = call "Read Manufacturer Data.vi"("Unit ID (A)"=w251, "error in"=w254, "VISA Session In"=w253) -> ("error out"=w262:errorcluster, "Manufacturer Info"=→"Manufacturer Info":string, "VISA Session Out"=w263:refnum<visa-resource-name>)  [unwired: 6 in]
            n43 = property on="COMPOSER gas 2" class="Ring (strict)"("StringsAndValues[]"=w249) -> ()  [unwired: 2 in, 2 out]
            n44 = property on="COMPOSER gas 3" class="Ring (strict)"("StringsAndValues[]"=w249) -> ()  [unwired: 2 in, 2 out]
            n45 = Unbundle By Name(w233) -> ("Setpoint"=→"Setpoint Units":string, "Totalizer"=→"Batch Units":string)
            n46 = property on="COMPOSER gas 4" class="Ring (strict)"("StringsAndValues[]"=w249) -> ()  [unwired: 2 in, 2 out]
            n47 = property on="COMPOSER gas 5" class="Ring (strict)"("StringsAndValues[]"=w249) -> ()  [unwired: 2 in, 2 out]
          }
          frame 2 {
            w279 = u16 0 items=["No controller"=0, "Volumetric Flow"=36, "Mass Flow"=37, "Absolute Pressure"=34, "Gauge Pressure"=38, "Differential Pressure"=39] ("Controller Select")
            # "Obtain digits to the left of the decimal\nand check if batching is available"
            # "Determine units for setpoint"
            # "initialize the enables/disables\nto current settings (to avoid \naccidental disables)"
            # "Obtain second set of options and initialize the respective controls/indicators"
            n48 = call "Batch Detect.vi"("Unit ID (A)"=w316, "error in"=w296, "VISA Session In"=w297) -> ("error out"=w326:errorcluster, "Batching available"=w308:bool, "VISA Session Out"=w325:refnum<visa-resource-name>)  [unwired: 6 in]
            n49 = Increment(x=w328) -> (x+1=w311:i32)
            n50 = call "Read Measurement Format.vi"("Unit ID (A)"=w316, "error in"=w326, "VISA Session In"=w325) -> ("error out"=w319:errorcluster, "Data Frame Format"=w321:T13, "VISA Session Out"=w320:refnum<visa-resource-name>)  [unwired: 6 in]
            n51 = Unbundle(w322) -> ("Enabled"=w313:T26, "Disabled and Grayed Out"=w314:T26)
            n52 = Unbundle(w321) -> ("Absolute Pressure"=w293:bool, "Gauge/Diff. Pressure"=w292:bool, "Barometric Pressure"=w291:bool, "Temperature"=w285:bool, "Volumetric"=w286:bool, "Mass"=w287:bool, "Valve Drive"=w284:bool, "Totalizer"=w283:bool, "Totalizer Timer"=w282:bool, "Totalizer Average Flow"=w288:bool, "Totalizer Peak Flow"=w281:bool, "Gas Selected"=w289:bool)  [unwired: 2 out]
            n53 = Or(x=w293, y=w292) -> (x .or. y?=w290:bool)
            n54 = Bundle(cluster=T20 {"Pressure(s)"=TRUE, "Temperature"=TRUE, "Volumetric"=TRUE, "Mass"=TRUE, "Totalizer Average Flow"=FALSE, "Gas Selected"=TRUE} ("Enables: \nData frame and Display"), "Pressure(s)"=w290, "Temperature"=w285, "Volumetric"=w286, "Mass"=w287, "Totalizer Average Flow"=w288, "Gas Selected"=w289) -> (w324:T20)
            n55 = Bundle(cluster=T2 {"Valve Drive"=FALSE, "Totalizer"=TRUE, "Totalizer Timer"=FALSE, "Totalizer Peak Flow"=FALSE, "Show Abs., Gauge\nand Baro. pressures"=FALSE} ("Enables: Data frame only"), "Valve Drive"=w284, "Totalizer"=w283, "Totalizer Timer"=w282, "Totalizer Peak Flow"=w281, "Show Abs., Gauge\nand Baro. pressures"=w291) -> (w280:T2)
            n56 = call "Read Controller Info.vi"("Unit ID (A)"=w316, "error in"=w319, "Software Version"=w299, "VISA Session In"=w320) -> ("error out"=w318:errorcluster, "Disabled Items\n(used with\"DisabledItems[]\" in the\nController Select property node)"=w277:i32[], "Controller Info out"=w298:T14, "VISA Session Out"=w317:refnum<visa-resource-name>)  [unwired: 4 in]
            n57 = Unbundle By Name(w298) -> ("Controller Full Scale"=→"(Full Scale)":dbl, "Controller Select"=w312:u16)
            n58 = property on="Serial and Display" class="Clust (strict)"("Value"=w324) -> ()  [unwired: 2 in, 2 out]
            n59 = property on="Serial Only" class="Clust (strict)"("Value"=w280) -> ()  [unwired: 2 in, 2 out]
            n60 = property on="Controller Select" class="Ring (strict)"("Disabled Items []"=w277) -> ()  [unwired: 2 in, 2 out]
            n61 = Not Equal?(x=w312, y=w279) -> (x != y?=w307:bool)
            n62 = And(x=w308, y=w307) -> (x .and. y?=w306:bool)
            n63 = Select(t=w313, s=w306, f=w314) -> (s? t:f=w327:T26)
            n64 = Select(t=w313, s=w307, f=w314) -> (s? t:f=w315:T26)
            n65 = property on="Batch Setpoint" class="DigNum (strict)"("DisabledEnum"=w327) -> ()  [unwired: 2 in, 2 out]
            n66 = property on="Setpoint" class="DigNum (strict)"("DisabledEnum"=w315) -> ()  [unwired: 2 in, 2 out]
          }
          frame 3 {
            # "Get Totalizer info and check which tare functions are allowable"
            # "Obtain the third set of options and initialize the respective controls/indicators"
            n67 = call "Flow and Pressure Function Check.vi"("Unit ID (A)"=w341, "error in"=w363, "Software Version"=w330, "VISA Session In"=w362) -> ("error out"=w359:errorcluster, "Flow Tare Enabled"=w352:bool, "Pressure Tare Enabled"=w351:bool, "VISA Session Out"=w358:refnum<visa-resource-name>)  [unwired: 4 in]
            n68 = Increment(x=w343) -> (x+1=w342:i32)
            n69 = Unbundle(w355) -> ("Enabled"=w338:T26, "Disabled and Grayed Out"=w337:T26)
            n70 = call "Read Totalizer Units and Decimals.vi"("Unit ID (A)"=w341, "error in"=w359, "Software Version"=w330, "VISA Session In"=w358) -> ("error out"=w346:errorcluster, "Totalizer"=w356:T10, "VISA Session Out"=w345:refnum<visa-resource-name>, "Totalizer decimal places"=w361:i32)  [unwired: 3 in, 1 out]
            "Totalizer" <- w356
            n71 = To Unsigned Byte Integer(number=w361) -> (unsigned 8bit integer=w360:u8)
            n72 = Select(t=w338, s=w351, f=w337) -> (s? t:f=w354:T26)
            n73 = Select(t=w338, s=w352, f=w337) -> (s? t:f=w353:T26)
            n74 = property on="Batch Setpoint" class="DigNum (strict)"("Precision"=w360) -> ()  [unwired: 2 in, 2 out]
            n75 = property on="Tare Pressure" class="Bool"("DisabledEnum"=w354) -> ()  [unwired: 2 in, 2 out]
            n76 = property on="Tare Flow" class="Bool"("DisabledEnum"=w353) -> ()  [unwired: 2 in, 2 out]
            n77 = Not Equal?(x=w356, y=T10."No Totalizer" ("Totalizer")) -> (x != y?=w349:bool)
            n78 = Select(t=w338, s=w349, f=w337) -> (s? t:f=w350:T26)
            n79 = property on="Reset Total" class="Bool"("DisabledEnum"=w350) -> ()  [unwired: 2 in, 2 out]
          }
          frame 4 {
            # "Initialize controller and tare options, and determine if they need to be disabled"
            # "Obtain the fourth set of options and initialize the respective controls/indicators"
            n80 = call "Read Tare Settings.vi"("Unit ID (A)"=w391, "error in"=w383, "VISA Session In"=w382) -> ("error out"=w376:errorcluster, "Tare Functions"=w390:T9, "VISA Session Out"=w377:refnum<visa-resource-name>)  [unwired: 6 in]
            n81 = Increment(x=w403) -> (x+1=w401:i32)
            n82 = Unbundle(w402) -> ("Enabled"=w386:T26, "Disabled and Grayed Out"=w385:T26)
            n83 = Unbundle(w390) -> ("Display"=w387:enum16{"None", "Pressure", "Volumetric"}, "External"=w388:T27, "Auto-Tare Delay [s]"=w389:dbl)
            n84 = Select(t=w386, s=w384, f=w385) -> (s? t:f=w365:T26)
            n85 = property on="Auto-Tare Delay [s]" class="DigNum (strict)"("Value"=w389, "DisabledEnum"=w365) -> ()  [unwired: 2 in, 2 out]
            n86 = property on="Display" class="Enum (strict)"("Value"=w387) -> ()  [unwired: 2 in, 2 out]
            n87 = property on="External" class="Enum (strict)"("Value"=w388) -> ()  [unwired: 2 in, 2 out]
            n88 = call "Read PID Info.vi"("VISA Session In"=w377, "error in"=w376, "Unit ID (A)"=w391) -> ("VISA Session Out"=w380:refnum<visa-resource-name>, "PID Settings"=w397:T28, "error out"=w381:errorcluster)  [unwired: 5 in]
            n89 = Unbundle(w397) -> ("PID Type"=w396:enum8{"PDF", "PD2I"}, "Valve Offset"=w395:i32, "P Gain"=w394:i32, "D Gain"=w393:i32, "I Gain"=w392:i32)  [unwired: 1 out]
            n90 = property on="PID Type" class="Enum (strict)"("Value"=w396, "DisabledEnum"=w365) -> ()  [unwired: 2 in, 2 out]
            n91 = property on="P Gain" class="DigNum (strict)"("Value"=w394, "DisabledEnum"=w365) -> ()  [unwired: 2 in, 2 out]
            n92 = property on="I Gain" class="DigNum (strict)"("Value"=w392, "DisabledEnum"=w365) -> ()  [unwired: 2 in, 2 out]
            n93 = property on="Valve \nOffset" class="DigNum (strict)"("Value"=w395, "DisabledEnum"=w365) -> ()  [unwired: 2 in, 2 out]
            n94 = property on="D Gain" class="DigNum (strict)"("Value"=w393, "DisabledEnum"=w365) -> ()  [unwired: 2 in, 2 out]
            n95 = call "Read Output Definitions and Controller Options.vi"("Unit ID (A)"=w391, "error in"=w381, "Software Version"=w368, "VISA Session In"=w380) -> ("error out"=w379:errorcluster, "Read-Only Options"=→"Read-Only Options":T8, "Read/Write Options"=w369:T1, "VISA Session Out"=w378:refnum<visa-resource-name>)  [unwired: 4 in]
            n96 = Unbundle(w369) -> ("Controller Select"=w364:u16, "SetPoint Source"=w366:enum8{"Serial", "Local", "Analog", "Unknown"}, "AutoTare"=w367:enum16{"Disabled", "Enabled"})
            n97 = property on="Controller Select" class="Ring (strict)"("Value"=w364, "DisabledEnum"=w365) -> ()  [unwired: 2 in, 2 out]
            n98 = property on="SetPoint Source" class="Enum (strict)"("Value"=w366, "DisabledEnum"=w365) -> ()  [unwired: 2 in, 2 out]
            n99 = property on="AutoTare" class="Enum (strict)"("Value"=w367, "DisabledEnum"=w365) -> ()  [unwired: 2 in, 2 out]
          }
          frame 5 {
            w429 = 60.0 ("Pressure")
            # "This VI can not tell if the range is bi-directional or 0 to (-) full scale. This is due to how those are handled in the software.\n As this does not affect the data output, it should not be an issue other than needing to use the auto-scale features of LabVIEW."
            # "Update the chart to have the proper full scales"
            n100 = call "Read Controllable Fullscale Values.vi"("Unit ID (A)"=w416, "error in"=w423, "Software Version"=w422, "VISA Session In"=w424) -> ("error out"=w418:errorcluster, "Fullscale"=w412:T29, "VISA Session Out"=w419:refnum<visa-resource-name>)  [unwired: 5 in]
            n101 = Unbundle By Name(w433) -> ("Controller Select"=w432:u16)
            n102 = Increment(x=w435) -> (x+1=w434:i32)
            n103 = call "Read Register.vi"("Unit ID (A)"=w416, "error in"=w418, "Register address"=u16 38, "VISA Session In"=w419) -> ("error out"=w420:errorcluster, "Register Value (I32)"=w414:i32, "VISA Session Out"=w421:refnum<visa-resource-name>)  [unwired: 5 in]
            n104 = Unbundle(w412) -> ("Absolute Pressure"=w410:dbl, "Gauge/Diff. Pressure"=w409:dbl, "Volumetric Flow"=w407:dbl, "Mass Flow"=w406:dbl)
            n105 = And(x=w414, y=1) -> (x .and. y?=w413:i32)
            n106 = Not Equal To 0?(x=w413) -> (x != 0?=w411:bool)
            n107 = Select(t=w410, s=w411, f=w409) -> (s? t:f=w408:dbl)
            n108 = Build Array(w408, w429, w407, w406, w429) -> (w430:dbl[])
            n109 = Unbundle By Name(w428) -> ("Chart: AutoScale"=w427:bool)
            n110 = for {
              tunnel: w432 -> [w456]
              tunnel: w430 -> [w451] mode=indexing
              tunnel: [w450] -> _
              i -> [w454]
              # "Set each plot's Y scale, sequentially"
              n111 = Equal?(x=4, y=w454) -> (x = y?=w452:bool)
              n112 = To Unsigned Long Integer(number=w454) -> (unsigned 32bit integer=w453:u32)
              n113 = case shown="True" w452 {
                tunnel: w456 -> [_ w463]
                tunnel: w453 -> [w460 w462]
                tunnel: w451 -> [w458 _]
                tunnel: [u32 0 ("Active Plot") w461] -> w450
                frame False {
                  # "Set the Y scale ranges"
                  n114 = property on="Chart" class="WFChart (strict)"("Active Plot"=w460, "YScale.Maximum"=w458, "YScale.Minimum"=0.0 ("Y Scale.Range:Minimum")) -> ()  [unwired: 2 in, 2 out]
                }
                frame True {
                  # "Associate the setpoint scale properly"
                  n115 = case shown="0, Default" w463 {
                    tunnel: [u32 0 ("Active Plot") u32 0 ("Active Plot") u32 1 ("Active Plot") u32 1 ("Active Plot")] -> w461
                    frame 0, Default {
                    }
                    frame 34, 38, 39 {
                      # "Get setpoint scale"
                    }
                    frame 36 {
                    }
                    frame 37 {
                    }
                  }
                  n116 = property on="Chart" class="WFChart (strict)"("Active Plot"=w462, "Plot.YScaleIdx"=w461) -> ()  [unwired: 2 in, 2 out]
                }
              }
            }
            n117 = case shown="True" w427 {
              frame False {
              }
              frame True {
                w444 = u8 2 ("Y Scale.Scale Fit")
                # "AutoScale is true"
                n118 = property on="Chart" class="WFChart (strict)"("Active Plot"=u32 0, "YScale.ScaleFit"=w444, "Active Plot"=u32 1, "YScale.ScaleFit"=w444, "Active Plot"=u32 2, "YScale.ScaleFit"=w444, "Active Plot"=u32 3, "YScale.ScaleFit"=w444, "Active Plot"=u32 4, "YScale.ScaleFit"=w444) -> ()  [unwired: 2 in, 2 out]
              }
            }
          }
          frame 6 {
            w479 = FALSE ("Visible")
            # "Generate Logging info, hide initialization notification, and re-enable updates to the front panel (and close the related references)"
            n119 = property on="Data Logging Options" class="Clust (strict)"() -> ("Value"=w468:T3)  [unwired: 2 in, 2 out]
            n120 = Increment(x=w473) -> (x+1=w474:i32)
            n121 = Unbundle By Name(w468) -> ("Log Data"=w471:bool)
            n122 = case shown="True" w471 {
              tunnel: ["" w501] -> w484
              frame False {
              }
              frame True {
                n123 = Get Date/Time In Seconds() -> (seconds since 1Jan1904=w507:timestamp)
                n124 = Format Date/Time String(time format string (%c)="%m-%d-%Y_%H-%M-%S", seconds (now)=w507) -> (date/time string=w506:string)  [unwired: 1 in]
                n125 = call <vilib>:"Application Directory.vi"() -> ("Application Directory"=w503:path)
                n126 = Format Date/Time String(time format string (%c)="%p", seconds (now)=w507) -> (date/time string=w505:string)  [unwired: 1 in]
                n127 = Path To String(path=w503) -> (string=w500:string)
                n128 = Concatenate Strings(w500, "\\Alicat Data Log_" ("string"), w506, "_" ("string"), w505, ".txt" ("string")) -> (w501:string)
              }
            }
            n129 = call "Data Logging_Generate Header.vi"("error in"=w486, "Include Units\nin Header (F)"=TRUE ("Include Units\nin Header (default is F)"), "Units of Measure Input"=w485, "Data Logging Options"=w468) -> ("error out"=w482:errorcluster, "Data Log Header"=w480:string)  [unwired: 6 in]
            n130 = String To Path(string=w484) -> (path=w483:path)
            n131 = case shown="True" w471 {
              tunnel: w483 -> [_ w518]
              tunnel: w482 -> [w511 w517]
              tunnel: [w511 w515] -> w481
              tunnel: w480 -> [_ w514]
              tunnel: [refnum<file> refnum ("refnum out") w513] -> w478
              tunnel: T21."replace or create" ("operation (0:open)") -> [_ w512]
              frame False {
              }
              frame True {
                n132 = Open/Create/Replace File(file path (use dialog)=w518, error in=w517, operation (0:open)=w512) -> (refnum out=w519:refnum<file>, error out=w516:errorcluster)  [unwired: 3 in, 1 out]
                n133 = Write to Text File(file (use dialog)=w519, text=w514, error in=w516) -> (refnum out=w513:refnum<file>, error out=w515:errorcluster)  [unwired: 1 in, 1 out]
              }
            }
            n134 = Unbundle(w491) -> ("Panel"=w489:refnum<vi>)  [unwired: 1 out]
            n135 = property on="Wait message" class="Clust (strict)"(error in=w481, "Visible"=w479) -> (error out=w490:errorcluster)  [unwired: 1 in, 1 out]
            n136 = property class="Pnl"(reference=w489, error in=w490, "DeferPanUpdts"=w479) -> (error out=w475:errorcluster)  [unwired: 1 out]
          }
          frame 7, Default {
            w541 = TRUE ("Data Changed")
            # "No incrementing, this is the data collection state"
            # "Update setpoint control\nto current value on 1st run"
            # "Acquire data"
            # "Data collection"
            n137 = Wait (ms)(milliseconds to wait="Time between \nreadings [ms]") -> ()  [unwired: 1 out]
            n138 = call "Read Measurements.vi"("error in"=w557, "Data Frame Format In"=w556, "Unit ID (A)"=w552, "VISA Session In"=w558) -> ("error out"=w550:errorcluster, "Data Frame Format Out"=w537:T13, "Data Cluster"=w572:T30, "VISA Session Out"=w551:refnum<visa-resource-name>, "Unknown Dataframe Info"=w553:bool, "Error/Overrange/Unknown String"=w521:string, "Error Present"=w554:bool, "Range Exceeded"=w533:bool)
            n139 = Or(x=w553, y=w554) -> (x .or. y?=w532:bool)
            n140 = Unbundle(w572) -> ("Absolute Pressure"=w559:dbl, "Gauge/Diff. Pressure"=w560:dbl, "Barometric Pressure"=w561:dbl, "Temperature"=w562:dbl, "Volumetric Flow"=w546:dbl, "Mass Flow"=w563:dbl, "Setpoint"=w536:dbl, "Valve Drive"=w564:dbl, "Totalizer"=w565:dbl, "[hr]"=w566:dbl, "[min]"=w567:dbl, "[sec]"=w568:dbl, "Totalizer Average Flow"=w569:dbl, "Totalizer Peak Flow"=w535:dbl, "Gas selected"=w534:string)
            n141 = Unbundle(w555) -> ("Abs. Pressure"=w531:string, "Gauge/Diff. Press."=w527:string, "Barometric Press."=w526:string, "Temperature"=w528:string, "Volume"=w525:string, "Mass"=w524:string, "Setpoint"=w522:string, "Valve Drive"=w520:string, "Totalizer"=w523:string, "Tot. Avg. Flow"=w529:string, "Tot. Peak Flow"=w530:string)  [unwired: 1 out]
            n142 = Bundle(cluster=w571, "Absolute Pressure"=w559, "Gauge/Diff. Pressure"=w560, "Barometric Pressure"=w561, "Temperature"=w562, "Volumetric Flow"=w546, "Mass Flow"=w563, "Setpoint"=w536, "Valve Drive"=w564, "Totalizer"=w565, "[h]"=w566, "[m]"=w567, "[s]"=w568, "Totalizer Average Flow"=w569, "Totalizer Peak Flow"=w535, "Gas selected"=w534, "Range Exceeded"=w533, "Error Present"=w532, "ERR/OVR Text"=w521, "Abs. Pressure"=w531, "Temperature 2"=w528, "Volume"=w525, "Mass"=w524, "Totalizer 2"=w523, "Valve Drive 2"=w520, "Gauge/Diff. Press."=w527, "Barometric Press."=w526, "Setpoint 2"=w522, "Tot. Avg. Flow"=w529, "Tot. Peak Flow"=w530) -> (w570:T15)
            n143 = case shown="False" w540 {
              tunnel: w536 -> [w573 _]
              frame False {
                n144 = property on="Setpoint" class="DigNum (strict)"("Value"=w573) -> ()  [unwired: 2 in, 2 out]
              }
              frame True {
              }
            }
          }
        }
        n145 = Select(t=0, s=w171, f=w173) -> (s? t:f=w172:i32)
      }
      event Panel Close? {
        w591 = TRUE ("Discard?")
        # "Discard a panel close command and force the program to end (forces references to be closed before exiting)"
        n146 = event-data() -> ()  [unwired: 1 in, 1 out]
        n147 = event-data("Discard?"=w591) -> ()  [unwired: 1 in, 1 out]
      }
      event "COM Port Settings.VISA Sesssion In": Value Change {
        # "Re-initialize VI"
        # "Close the VISA session and re-initialize it with the new COM port value. Then, it resets the state to 0 to initialize the device"
        n148 = event-data() -> ("NewVal"=w592:refnum<visa-resource-name>)  [unwired: 1 in]
        n149 = VISA Close(VISA resource name=w604, error in (no error)=w605) -> (error out=w606:errorcluster)
        n150 = property on="Baud Rate" class="Enum (strict)"() -> ("Value"=w593:T31)  [unwired: 2 in, 2 out]
        n151 = Bundle(cluster=T12 {"Unit ID"="A", "Baud Rate"=enum."19200", "VISA Sesssion In"="COM1"} ("Communication Settings"), "Unit ID"="A", "Baud Rate"=w593, "VISA Sesssion In"=w592) -> (w595:T12)
        n152 = call "COM Port Initialization.vi"("error in (no error)"=w606, "Communication Settings"=w595) -> ("error out"=w609:errorcluster, "VISA Session Out"=w608:refnum<visa-resource-name>)  [unwired: 8 in]
      }
      event "COM Port Settings.Baud Rate": Value Change {
        # "Re-initialize VI"
        # "Changes the baud rate to match updated value, then it resets the state to 0 to initialize the device"
        n153 = event-data() -> ("NewVal"=w625:T31)  [unwired: 1 in]
        n154 = case shown="\"38400\"" w625 {
          tunnel: [u32 2400 ("Serial Settings:Baud Rate") u32 9600 ("Serial Settings:Baud Rate") u32 19200 ("Serial Settings:Baud Rate") u32 38400 ("Serial Settings:Baud Rate") u32 57600 ("Serial Settings:Baud Rate") u32 11520 ("Serial Settings:Baud Rate") u32 19200 ("Serial Settings:Baud Rate")] -> w624
          frame "2400", Default {
          }
          frame "9600" {
          }
          frame "19200" {
          }
          frame "38400" {
          }
          frame "57600" {
          }
          frame "115200" {
          }
          frame "Unknown" {
          }
        }
        n155 = property class="Serial Instr"(reference=w627, error in=w629, "Baud"=w624) -> (reference out=w626:refnum<visa-resource-name>, error out=w628:errorcluster)
      }
      event "COM Port Settings.Unit ID": Value Change {
        # "Re-initialize VI"
        # "Changes the unit ID to the new value, and then it resets the state to 0 to initialize the device"
        n156 = event-data() -> ("NewVal"=w652:string)  [unwired: 1 in]
      }
      event "Tare Flow": Value Change {
        # "Reset to 0 if\ncomm error\nis present"
        # "Executes the flow tare sub-VI and checks to make sure that the communication to the unit is still established"
        n157 = event-data() -> ()  [unwired: 1 in, 1 out]
        n158 = call "Tare Flow.vi"("Unit ID (A)"=w669, "error in"=w673, "VISA Session In"=w670) -> ("error out"=w672:errorcluster, "VISA Session Out"=w671:refnum<visa-resource-name>)  [unwired: 7 in]
        n159 = Select(t=0, s=w672, f=w674) -> (s? t:f=w675:i32)
      }
      event "Tare Pressure": Value Change {
        # "Reset to 0 if\ncomm error\nis present"
        # "Executes the pressure tare sub-VI and checks to make sure that the communication to the unit is still established"
        n160 = event-data() -> ()  [unwired: 1 in, 1 out]
        n161 = call "Tare Pressure.vi"("Unit ID (A)"=w690, "error in"=w694, "VISA Session In"=w691) -> ("error out"=w693:errorcluster, "VISA Session Out"=w692:refnum<visa-resource-name>)  [unwired: 7 in]
        n162 = Select(t=0, s=w693, f=w695) -> (s? t:f=w696:i32)
      }
      event "Tare AP Sensor": Value Change {
        # "Reset to 0 if\ncomm error\nis present"
        # "Executes the pressure tare sub-VI and checks to make sure that the communication to the unit is still established"
        n163 = event-data() -> ()  [unwired: 1 in, 1 out]
        n164 = call "Tare AP Sensor with Internal Barometer.vi"("Unit ID (A)"=w711, "error in"=w715, "VISA Session In"=w712) -> ("error out"=w714:errorcluster, "VISA Session Out"=w713:refnum<visa-resource-name>)  [unwired: 7 in]
        n165 = Select(t=0, s=w714, f=w716) -> (s? t:f=w717:i32)
      }
      event "Reset Total": Value Change {
        # "Reset to 0 if\ncomm error\nis present"
        # "Executes the Totalizer reset sub-VI and checks to make sure that the communication to the unit is still established"
        n166 = event-data() -> ()  [unwired: 1 in, 1 out]
        n167 = call "Reset Totalizer.vi"("Unit ID (A)"=w732, "error in"=w736, "VISA Session In"=w733) -> ("error out"=w735:errorcluster, "VISA Session Out"=w734:refnum<visa-resource-name>)  [unwired: 6 in, 1 out]
        n168 = Select(t=0, s=w735, f=w737) -> (s? t:f=w738:i32)
      }
      event "Tare Options": Value Change {
        # "Reset to 0 if\ncomm error\nis present"
        # "Writes the new tare settings and checks to make sure that the communication to the unit is still established"
        n169 = event-data() -> ()  [unwired: 1 in, 1 out]
        n170 = call "Write Tare Settings.vi"("Unit ID (A)"=w753, "error in"=w755, "Tare Functions"="Tare Options", "VISA Session In"=w758) -> ("error out"=w756:errorcluster, "VISA Session Out"=w757:refnum<visa-resource-name>)  [unwired: 6 in]
        n171 = Select(t=0, s=w756, f=w759) -> (s? t:f=w760:i32)
      }
      event "Gas Select": Value Change {
        # "Reset to 0 if\ncomm error\nis present"
        # "Writes the new gas selection and checks to make sure that the communication to the unit is still established"
        n172 = event-data() -> ()  [unwired: 1 in, 1 out]
        n173 = call "Write Gas Selection.vi"("Unit ID (A)"=w776, "error in"=w777, "Gas Number"="Gas Select", "VISA Session In"=w780) -> ("error out"=w778:errorcluster, "VISA Session Out"=w779:refnum<visa-resource-name>)  [unwired: 6 in]
        n174 = Select(t=0, s=w778, f=w781) -> (s? t:f=w782:i32)
      }
      event "Read/Write Options": Value Change {
        # "Disallow changing of control variable \nto \"no controller\" if it is a controller.\nAlso, discard invalid choices and notify user"
        # "Reset to 0 if\ncomm error\nis present"
        # "Writes the new controller options (if allowable) and checks to make sure that the communication to the unit is still established"
        n175 = event-data() -> ()  [unwired: 1 in, 6 out]
        n176 = Unbundle By Name(w811) -> ("Controller Select"=w803:u16)
        n177 = Unbundle("Read/Write Options") -> ("Controller Select"=w804:u16, "SetPoint Source"=w810:enum8{"Serial", "Local", "Analog", "Unknown"}, "AutoTare"=w809:enum16{"Disabled", "Enabled"})
        n178 = call "Controller Select_Check Validity.vi"("Software Version"=w792, "Controller?"=w798, "Unit ID (A)"=w797, "error in"=w822, "Controller Select_Old"=w803, "Controller Select_New"=w804, "VISA Session In"=w802) -> ("error out"=w800:errorcluster, "Invalid selection"=w799:bool, "Validated Controller Select"=w790:u16, "VISA Session Out"=w801:refnum<visa-resource-name>)  [unwired: 1 in]
        n179 = Bundle(cluster="Read/Write Options", "Controller Select"=w790, "SetPoint Source"=w810, "AutoTare"=w809) -> (w808:T1)
        n180 = call "Write Controller Options.vi"("Unit ID (A)"=w797, "error in"=w800, "Software Version"=w792, "Read/Write Options"=w808, "VISA Session In"=w801) -> ("error out"=w812:errorcluster, "VISA Session Out"=w813:refnum<visa-resource-name>)  [unwired: 5 in]
        n181 = case shown="0, Default" w790 {
          tunnel: [u32 0 ("Active Plot") u32 0 ("Active Plot") u32 1 ("Active Plot") u32 1 ("Active Plot")] -> w791
          frame 0, Default {
          }
          frame 34, 38, 39 {
            # "Get setpoint scale"
          }
          frame 36 {
          }
          frame 37 {
          }
        }
        n182 = property on="Chart" class="WFChart (strict)"("Active Plot"=u32 4, "Plot.YScaleIdx"=w791) -> ()  [unwired: 2 in, 2 out]
        n183 = call "Display Message to User4"("Enable"=w799) -> ()  [unwired: 9 in, 2 out]
        n184 = Select(t=0, s=w812, f=w814) -> (s? t:f=w815:i32)
      }
      event "PID Settings.P Gain", "PID Settings.D Gain", "PID Settings.I Gain": Value Change {
        # "Reset to 0 if\ncomm error\nis present"
        # "Writes the new PID settings and checks to make sure that the communication to the unit is still established"
        n185 = event-data() -> ()  [unwired: 1 in, 1 out]
        n186 = Unbundle("PID Settings") -> ("P Gain"=w840:i32, "D Gain"=w839:i32, "I Gain"=w838:i32)  [unwired: 2 out]
        n187 = Bundle(cluster=T22 {"P Gain"=0, "D Gain"=0, "I Gain"=0} ("PID Gain Settings"), "P Gain"=w840, "D Gain"=w839, "I Gain"=w838) -> (w842:T22)
        n188 = call "Write PID Gains.vi"("VISA Session In"=w843, "PID Gain Settings"=w842, "error in"=w844, "Unit ID (A)"=w835) -> ("VISA Session Out"=w837:refnum<visa-resource-name>, "error out"=w836:errorcluster)  [unwired: 5 in]
        n189 = Select(t=0, s=w836, f=w845) -> (s? t:f=w846:i32)
      }
      event "PID Settings.PID Type", "PID Settings.Valve \nOffset": Value Change {
        # "Reset to 0 if\ncomm error\nis present"
        # "Writes the new PID settings and checks to make sure that the communication to the unit is still established"
        n190 = event-data() -> ()  [unwired: 1 in, 6 out]
        n191 = property on="PID Settings" class="Clust (strict)"() -> ("Value"=w861:T7)  [unwired: 2 in, 2 out]
        n192 = Unbundle(w861) -> ("PID Type"=w866:enum8{"PDF", "PD2I"}, "Valve \nOffset"=w865:i32)  [unwired: 3 out]
        n193 = Bundle(cluster=T23 {"PID Type"=enum."PDF", "Valve Offset"=0} ("PID Loop Settings"), "PID Type"=w866, "Valve Offset"=w865) -> (w864:T23)
        n194 = call "Write PID Settings.vi"("VISA Session In"=w863, "PID Loop Settings"=w864, "error in"=w862, "Unit ID (A)"=w868) -> ("VISA Session Out"=w870:refnum<visa-resource-name>, "error out"=w869:errorcluster)  [unwired: 5 in]
        n195 = Select(t=0, s=w869, f=w871) -> (s? t:f=w872:i32)
      }
      event "COMPOSER gas mix input.Create COMPOSER Mix": Value Change {
        # "Create COMPOSER mix, then re-populate gas select lists"
        # "Reset to 0 if\ncomm error\nis present"
        # "Writes the desired COMPOSER mix (if possible), and checks to make sure that the communication to the unit is still established"
        n196 = event-data() -> ()  [unwired: 1 in, 6 out]
        n197 = Unbundle("COMPOSER gas mix input") -> ("Mix % 1"=w897:dbl, "Include # 1"=w898:bool, "Mix % 2"=w899:dbl, "Include # 2"=w900:bool, "Mix % 3"=w901:dbl, "Include # 3"=w902:bool, "Mix % 4"=w904:dbl, "Include # 4"=w903:bool, "Mix % 5"=w905:dbl, "Include # 5"=w906:bool, "COMPOSER gas 1"=w911:u16, "COMPOSER gas 2"=w910:u16, "COMPOSER gas 3"=w909:u16, "COMPOSER gas 4"=w908:u16, "COMPOSER gas 5"=w907:u16, "Mix #"=w895:u16, "Mix name"=w894:string)  [unwired: 3 out]
        n198 = Bundle(cluster=T24 {"Gas # 1"=236, "Mix % 1"=0.0, "Include # 1"=FALSE, "Gas # 2"=0, "Mix % 2"=0.0, "Include # 2"=FALSE, "Gas # 3"=0, "Mix % 3"=0.0, "Include # 3"=FALSE, "Gas # 4"=0, "Mix % 4"=0.0, "Include # 4"=FALSE, "Gas # 5"=0, "Mix % 5"=0.0, "Include # 5"=FALSE} ("COMPOSER gas mix input"), "Gas # 1"=w911, "Mix % 1"=w897, "Include # 1"=w898, "Gas # 2"=w910, "Mix % 2"=w899, "Include # 2"=w900, "Gas # 3"=w909, "Mix % 3"=w901, "Include # 3"=w902, "Gas # 4"=w908, "Mix % 4"=w904, "Include # 4"=w903, "Gas # 5"=w907, "Mix % 5"=w905, "Include # 5"=w906) -> (w896:T24)
        n199 = call "Write COMPOSER Gas Mix.vi"("Gas mix name"=w894, "Unit ID (A)"=w884, "error in"=w914, "Gas # to store mix as"=w895, "COMPOSER gas mix input"=w896, "VISA Session In"=w915) -> ("error out"=w886:errorcluster, "Completion text"=w893:string, "VISA Session Out"=w887:refnum<visa-resource-name>)  [unwired: 3 in]
        n200 = property on="Completion\ntext" class="Str"("Value"=w893) -> ()  [unwired: 2 in, 2 out]
        n201 = call "Read Gas List.vi"("Unit ID (A)"=w884, "error in"=w886, "VISA Session In"=w887) -> ("error out"=w880:errorcluster, "Gas Selection: Strings and Values"=w881:cluster{"Gas Name":string, "Gas number":u16}[], "VISA Session Out"=w885:refnum<visa-resource-name>)  [unwired: 5 in, 1 out]
        n202 = property on="Gas Select" class="Ring (strict)"("StringsAndValues[]"=w881) -> ()  [unwired: 2 in, 2 out]
        n203 = property on="COMPOSER gas 1" class="Ring (strict)"("StringsAndValues[]"=w881) -> ()  [unwired: 2 in, 2 out]
        n204 = property on="COMPOSER gas 2" class="Ring (strict)"("StringsAndValues[]"=w881) -> ()  [unwired: 2 in, 2 out]
        n205 = property on="COMPOSER gas 3" class="Ring (strict)"("StringsAndValues[]"=w881) -> ()  [unwired: 2 in, 2 out]
        n206 = property on="COMPOSER gas 4" class="Ring (strict)"("StringsAndValues[]"=w881) -> ()  [unwired: 2 in, 2 out]
        n207 = property on="COMPOSER gas 5" class="Ring (strict)"("StringsAndValues[]"=w881) -> ()  [unwired: 2 in, 2 out]
        n208 = Select(t=0, s=w880, f=w916) -> (s? t:f=w917:i32)
      }
      event "Read Register": Value Change {
        w933 = "%d" ("format string")
        # "Reset to 0 if\ncomm error\nis present"
        # "Reads desired register and displays it. Also checks to make sure that the communication to the unit is still established"
        n209 = event-data() -> ()  [unwired: 1 in, 6 out]
        n210 = Format Into String(format string=w933, initial string="R", "Reg. to read") -> (resulting string=w936:string)  [unwired: 1 in, 1 out]
        n211 = call "Read Register.vi"("Unit ID (A)"=w940, "error in"=w941, "Register address"="Reg. to read", "VISA Session In"=w944) -> ("error out"=w942:errorcluster, "Register Value (I32)"=w938:i32, "VISA Session Out"=w943:refnum<visa-resource-name>)  [unwired: 5 in]
        n212 = Concatenate Strings(w936, " = " ("string")) -> (w934:string)
        n213 = Format Into String(format string=w933, initial string=w934, w938) -> (resulting string=→"Register value":string)  [unwired: 1 in, 1 out]
        n214 = Select(t=0, s=w942, f=w945) -> (s? t:f=w946:i32)
      }
      event "Log Register Values": Value Change {
        # "Reset to 0 if\ncomm error\nis present"
        # "Logs the current register values to a text file in the folder containing this VI. Also checks to make sure that the communication to the unit is still established"
        n215 = event-data() -> ()  [unwired: 1 in, 6 out]
        n216 = call "Log Current Register Values.vi"("Unit ID (A)"=w970, "error in"=w971, "VISA Session In"=w973) -> ("error out"=w960:errorcluster, "VISA Session Out"=w972:refnum<visa-resource-name>)  [unwired: 7 in]
        n217 = Get Date/Time String(want seconds? (F)=TRUE) -> (date string=w966:string, time string=w965:string)  [unwired: 2 in]
        n218 = Concatenate Strings(w966, ", " ("string"), w965) -> (w961:string)
        n219 = Concatenate Strings("Register log saved in VI folder." ("Message"), w961) -> (w963:string)
        n220 = call "Display Message to User"("error in (no error)"=w960, "Message"=w963) -> ("error out"=w959:errorcluster)  [unwired: 8 in, 1 out]
        n221 = Select(t=0, s=w959, f=w974) -> (s? t:f=w975:i32)
      }
      event "Batch Setpoint": Value Change {
        # "Reset to 0 if\ncomm error\nis present"
        # "Writes a new batch setpoint and checks to make sure that the communication to the unit is still established"
        n222 = event-data() -> ()  [unwired: 1 in, 1 out]
        n223 = call "Legacy Detector.vi"("Unit ID (A)"=w983, "error in"=w987, "VISA Session In"=w988) -> ("error out"=w986:errorcluster, "Legacy Status"=w984:u8, "VISA Session Out"=w985:refnum<visa-resource-name>)  [unwired: 6 in]
        n224 = call "Write Batch Setpoint.vi"("Unit ID (A)"=w983, "error in"=w986, "Batch SetPoint"="Batch Setpoint", "Legacy Status"=w984, "VISA Session In"=w985) -> ("error out"=w996:errorcluster, "VISA Session Out"=w998:refnum<visa-resource-name>)  [unwired: 5 in]
        n225 = Select(t=0, s=w996, f=w999) -> (s? t:f=w1000:i32)
      }
      event "Setpoint": Value Change {
        # "Reset to 0 if\ncomm error\nis present"
        # "Writes new setpoint if different from old setpoint, then parses the returned data frame and checks to make sure that the communication to the unit is still established"
        n226 = event-data() -> ("NewVal"=w1009:dbl)  [unwired: 1 in]
        n227 = call "Write SetPoint.vi"("Setpoint"=w1009, "Previous Setpoint"=w1062, "Unit ID (A)"=w1015, "error in"=w1064, "Software Version"=w1008, "Controller Info out"=w1057, "VISA Session In"=w1065) -> ("error out"=w1060:errorcluster, "Data frame returned"=w1012:string, "Controller Info out"=w1056:T14, "VISA Session Out"=w1017:refnum<visa-resource-name>)  [unwired: 1 in]
        n228 = call "Parse Data Frame.vi"("VISA Session In"=w1017, "Unit ID (A)"=w1015, "Data Frame Input"=w1012, "Data Frame Format In"=w1011, "error in"=w1060, "Offset (2 if polling, 0 if streaming)"=u32 2) -> ("Range Exceeded"=w1019:bool, "Error/Overrange/Unknown String"=w1020:string, "VISA Session Out"=w1016:refnum<visa-resource-name>, "Data Cluster"=w1023:T30, "Data Frame Format Out"=w1010:T13, "Error Present"=w1058:bool, "Unknown Dataframe Info"=w1059:bool, "error out"=w1055:errorcluster)  [unwired: 2 in]
        n229 = Or(x=w1059, y=w1058) -> (x .or. y?=w1018:bool)
        n230 = Unbundle(w1023) -> ("Absolute Pressure"=w1038:dbl, "Gauge/Diff. Pressure"=w1039:dbl, "Barometric Pressure"=w1040:dbl, "Temperature"=w1041:dbl, "Volumetric Flow"=w1037:dbl, "Mass Flow"=w1042:dbl, "Setpoint"=w1036:dbl, "Valve Drive"=w1043:dbl, "Totalizer"=w1044:dbl, "[hr]"=w1045:dbl, "[min]"=w1046:dbl, "[sec]"=w1047:dbl, "Totalizer Average Flow"=w1048:dbl, "Totalizer Peak Flow"=w1035:dbl, "Gas selected"=w1034:string)
        n231 = Unbundle(w1022) -> ("Abs. Pressure"=w1033:string, "Gauge/Diff. Press."=w1029:string, "Barometric Press."=w1028:string, "Temperature"=w1030:string, "Volume"=w1027:string, "Mass"=w1026:string, "Setpoint"=w1024:string, "Valve Drive"=w1021:string, "Totalizer"=w1025:string, "Tot. Avg. Flow"=w1031:string, "Tot. Peak Flow"=w1032:string)  [unwired: 1 out]
        n232 = Bundle(cluster=w1014, "Absolute Pressure"=w1038, "Gauge/Diff. Pressure"=w1039, "Barometric Pressure"=w1040, "Temperature"=w1041, "Volumetric Flow"=w1037, "Mass Flow"=w1042, "Setpoint"=w1036, "Valve Drive"=w1043, "Totalizer"=w1044, "[h]"=w1045, "[m]"=w1046, "[s]"=w1047, "Totalizer Average Flow"=w1048, "Totalizer Peak Flow"=w1035, "Gas selected"=w1034, "Range Exceeded"=w1019, "Error Present"=w1018, "ERR/OVR Text"=w1020, "Abs. Pressure"=w1033, "Temperature 2"=w1030, "Volume"=w1027, "Mass"=w1026, "Totalizer 2"=w1025, "Valve Drive 2"=w1021, "Gauge/Diff. Press."=w1029, "Barometric Press."=w1028, "Setpoint 2"=w1024, "Tot. Avg. Flow"=w1031, "Tot. Peak Flow"=w1032) -> (w1013:T15)
        n233 = property on="Time between \nreadings [ms]" class="DigNum (strict)"() -> ("Value"=w1052:u32)  [unwired: 2 in, 2 out]
        n234 = Wait (ms)(milliseconds to wait=w1052) -> ()  [unwired: 1 out]
        n235 = Select(t=0, s=w1055, f=w1066) -> (s? t:f=w1067:i32)
      }
      event "Serial and Display", "Serial Only": Value Change {
        # "If the requested data frame alteration is not possible, the change will\nbe rejected and the user will be notified."
        # "Reset to 0 if\ncomm error\nis present"
        # "Writes new data frame enables (if allowed), returns the new data frame format cluster, and checks to make sure that the communication to the unit is still established"
        n236 = event-data() -> ()  [unwired: 1 in, 6 out]
        n237 = call "Write Data Frame Options.vi"("Unit ID (A)"=w1105, "error in"=w1111, "Enables: Data frame only"="Serial Only", "Enables: \nData frame and Display"="Serial and Display", "VISA Session In"=w1112) -> ("error out"=w1107:errorcluster, "VISA Session Out"=w1106:refnum<visa-resource-name>)  [unwired: 5 in]
        n238 = call "Read Measurement Format.vi"("Unit ID (A)"=w1105, "error in"=w1107, "VISA Session In"=w1106) -> ("error out"=w1088:errorcluster, "Data Frame Format"=w1103:T13, "VISA Session Out"=w1108:refnum<visa-resource-name>)  [unwired: 6 in]
        n239 = Unbundle(w1103) -> ("Absolute Pressure"=w1083:bool, "Gauge/Diff. Pressure"=w1084:bool, "Barometric Pressure"=w1080:bool, "Temperature"=w1081:bool, "Volumetric"=w1079:bool, "Mass"=w1078:bool, "Valve Drive"=w1075:bool, "Totalizer"=w1074:bool, "Totalizer Timer"=w1073:bool, "Totalizer Average Flow"=w1077:bool, "Totalizer Peak Flow"=w1072:bool, "Gas Selected"=w1076:bool)  [unwired: 2 out]
        n240 = Or(x=w1083, y=w1084) -> (x .or. y?=w1082:bool)
        n241 = Bundle(cluster=T25 {"Pressure"=TRUE, "Temperature"=TRUE, "Volumetric"=TRUE, "Mass"=TRUE, "Totalizer Average Flow"=FALSE, "Gas Selected"=TRUE} ("Serial and Display"), "Pressure"=w1082, "Temperature"=w1081, "Volumetric"=w1079, "Mass"=w1078, "Totalizer Average Flow"=w1077, "Gas Selected"=w1076) -> (w1101:T25)
        n242 = Bundle(cluster=T2 {"Valve Drive"=FALSE, "Totalizer"=TRUE, "Totalizer Timer"=FALSE, "Totalizer Peak Flow"=FALSE, "Show Abs., Gauge\nand Baro. pressures"=FALSE} ("Serial Only"), "Valve Drive"=w1075, "Totalizer"=w1074, "Totalizer Timer"=w1073, "Totalizer Peak Flow"=w1072, "Show Abs., Gauge\nand Baro. pressures"=w1080) -> (w1071:T2)
        n243 = property on="Serial and Display" class="Clust (strict)"("Value"=w1101) -> ()  [unwired: 2 in, 2 out]
        n244 = property on="Serial Only" class="Clust (strict)"("Value"=w1071) -> ()  [unwired: 2 in, 2 out]
        n245 = Not Equal?(x="Serial and Display", y=w1101) -> (x != y?=w1098:T32)
        n246 = Not Equal?(x=w1071, y="Serial Only") -> (x != y?=w1091:T2)
        n247 = Cluster To Array(cluster=w1091) -> (array=w1093:bool[])
        n248 = Cluster To Array(cluster=w1098) -> (array=w1094:bool[])
        n249 = Build Array(w1094, w1093) -> (w1092:bool[][])
        n250 = Boolean To (0,1)(Boolean=w1092) -> (0, 1=w1097:i16[][])
        n251 = Add Array Elements(numeric array=w1097) -> (sum=w1095:i16)
        n252 = Not Equal To 0?(x=w1095) -> (x != 0?=w1096:bool)
        n253 = call "Display Message to User3"("Enable"=w1096) -> ()  [unwired: 9 in, 2 out]
        n254 = Select(t=0, s=w1088, f=w1113) -> (s? t:f=w1114:i32)
      }
      event "Chart: Pressure", "Chart: Temperature", "Chart: Volumetric", "Chart: Mass Flow", "Chart: Graphing", "Chart: Setpoint": Value Change {
        # "Reset to 0 if\ncomm error\nis present"
        # "Adjusts what variables are displayed in the chart, and checks to make sure that the communication to the unit is still established"
        n255 = event-data() -> ()  [unwired: 1 in, 6 out]
        n256 = property on="Chart" class="WFChart (strict)"("Active Plot"=u32 0, "Plot.Visible?"="Chart: Pressure", "Active Plot"=u32 1, "Plot.Visible?"="Chart: Temperature", "Active Plot"=u32 2, "Plot.Visible?"="Chart: Volumetric", "Active Plot"=u32 3, "Plot.Visible?"="Chart: Mass Flow", "Active Plot"=u32 4, "Plot.Visible?"="Chart: Setpoint") -> ()  [unwired: 2 in, 2 out]
        n257 = Select(t=0, s=w1139, f=w1142) -> (s? t:f=w1143:i32)
      }
      event "Chart: AutoScale": Value Change {
        # "Reset to 0 if\ncomm error\nis present"
        # "Toggles the autoscaling depending on the boolean control and checks to make sure that the communication to the unit is still established"
        n258 = event-data() -> ()  [unwired: 1 in, 6 out]
        n259 = case shown="True" "Chart: AutoScale" {
          frame False {
            w1170 = u8 0 ("Y Scale.Scale Fit")
            # "Turn off auto-scaling"
            n260 = property on="Chart" class="WFChart (strict)"("Active Plot"=u32 0, "YScale.ScaleFit"=w1170, "Active Plot"=u32 1, "YScale.ScaleFit"=w1170, "Active Plot"=u32 2, "YScale.ScaleFit"=w1170, "Active Plot"=u32 3, "YScale.ScaleFit"=w1170, "Active Plot"=u32 4, "YScale.ScaleFit"=w1170) -> ()  [unwired: 2 in, 2 out]
          }
          frame True {
            w1176 = u8 2 ("Y Scale.Scale Fit")
            # "AutoScale is true"
            n261 = property on="Chart" class="WFChart (strict)"("Active Plot"=u32 0, "YScale.ScaleFit"=w1176, "Active Plot"=u32 1, "YScale.ScaleFit"=w1176, "Active Plot"=u32 2, "YScale.ScaleFit"=w1176, "Active Plot"=u32 3, "YScale.ScaleFit"=w1176, "Active Plot"=u32 4, "YScale.ScaleFit"=w1176) -> ()  [unwired: 2 in, 2 out]
          }
        }
        n262 = Select(t=0, s=w1159, f=w1162) -> (s? t:f=w1163:i32)
      }
      event "Chart: Manual Scale Adjust": Value Change {
        w1198 = u8 0 ("Y Scale.Scale Fit")
        # "Disable auto-scaling, then go through a menu to set the new scales"
        # "Reset to 0 if\ncomm error\nis present"
        # "Toggles the autoscaling depending on the boolean control and checks to make sure that the communication to the unit is still established"
        n263 = event-data() -> ()  [unwired: 1 in, 1 out]
        n264 = property on="Chart" class="WFChart (strict)"(error in=w1197, "Active Plot"=u32 0, "YScale.ScaleFit"=w1198, "Active Plot"=u32 1, "YScale.ScaleFit"=w1198, "Active Plot"=u32 2, "YScale.ScaleFit"=w1198, "Active Plot"=u32 3, "YScale.ScaleFit"=w1198, "Active Plot"=u32 4, "YScale.ScaleFit"=w1198) -> (error out=w1189:errorcluster)  [unwired: 1 in, 1 out]
        n265 = call <vilib>:"Three Button Dialog.vi"("Allow user to close window? (TRUE)"=FALSE, "Window Title (\"\")"="Scale Adjustment Options" ("Window Title (\"\")"), "Right Button Text (\"Cancel\")"="Cancel" ("Left Button Text (\"Yes\")"), "Center Button Text (\"No\")"="Fit scales to current data" ("Left Button Text (\"Yes\")"), "Left Button Text (\"Yes\")"="Adjust scales manually" ("Left Button Text (\"Yes\")"), "message"="Adjust scales manually, or fit scales to current data?") -> ("Which Button?"=w1190:T33)  [unwired: 5 in]
        n266 = case shown="\"Left Button\", Default" w1190 {
          tunnel: w1189 -> [w1219 w1229 w1236]
          tunnel: [w1219 w1228 w1236] -> w1187
          tunnel: w1183 -> [w1218 _ _]
          frame "Left Button", Default {
            # "Adjust scales manually"
            n267 = call "Scale Adjustment Menu.vi"("Data Frame Format"=w1218) -> ("Scale Minimum"=w1221:dbl, "Scale Maximum"=w1222:dbl, "Active Y scale"=w1223:u32, "Request Cancelled"=w1220:bool)  [unwired: 6 in, 1 out]
            n268 = case shown="False" w1220 {
              tunnel: w1223 -> [w1224 _]
              tunnel: w1222 -> [w1227 _]
              tunnel: w1221 -> [w1226 _]
              frame False {
                # "Adjust scales if false"
                n269 = To Long Integer(number=w1224) -> (32bit integer=w1225:i32)
                n270 = property on="Chart" class="WFChart (strict)"("ActYScl"=w1225, "YScale.Maximum"=w1227, "YScale.Minimum"=w1226) -> ()  [unwired: 2 in, 2 out]
              }
              frame True {
                # "request was aborted"
              }
            }
          }
          frame "Center Button" {
            w1230 = u8 1 ("Y Scale.Scale Fit")
            # "Fit scales to current data"
            n271 = property on="Chart" class="WFChart (strict)"(error in=w1229, "Active Plot"=u32 0, "YScale.ScaleFit"=w1230, "Active Plot"=u32 1, "YScale.ScaleFit"=w1230, "Active Plot"=u32 2, "YScale.ScaleFit"=w1230, "Active Plot"=u32 3, "YScale.ScaleFit"=w1230, "Active Plot"=u32 4, "YScale.ScaleFit"=w1230) -> (error out=w1228:errorcluster)  [unwired: 1 in, 1 out]
          }
          frame "Right Button" {
            # "Request was aborted"
          }
        }
        n272 = property on="Chart: AutoScale" class="Bool (strict)"(error in=w1187, "Value"=FALSE ("Chart: AutoScale")) -> (error out=w1188:errorcluster)  [unwired: 1 in, 1 out]
        n273 = Select(t=0, s=w1188, f=w1210) -> (s? t:f=w1211:i32)
      }
      event "Data Logging Options": Value Change {
        # "Close current data file"
        # "Update the Logging options control with the valid options\n(essentially: throw out bad selections and notify the user)"
        # "Checks validity of choices and disables them if invalid. This also ensures that future data logging calls are using valid data"
        # "Reset to 0 if\ncomm error\nis present"
        # "Closes previously opened file (if applicable), opens a new one, and checks to make sure that the communication to the unit is still established"
        n274 = event-data() -> ()  [unwired: 1 in, 1 out]
        n275 = case shown="True" w1241 {
          tunnel: w1244 -> [_ w1273]
          tunnel: w1243 -> [w1270 w1272]
          tunnel: [w1270 w1271] -> w1242
          frame False {
          }
          frame True {
            n276 = Close File(refnum=w1273, error in=w1272) -> (error out=w1271:errorcluster)  [unwired: 1 out]
          }
        }
        n277 = Unbundle By Name("Data Logging Options") -> ("Log Data"=w1245:bool)
        n278 = case shown="True" w1245 {
          tunnel: ["" w1287] -> w1258
          frame False {
          }
          frame True {
            n279 = Get Date/Time In Seconds() -> (seconds since 1Jan1904=w1293:timestamp)
            n280 = Format Date/Time String(time format string (%c)="%m-%d-%Y_%H-%M-%S", seconds (now)=w1293) -> (date/time string=w1292:string)  [unwired: 1 in]
            n281 = call <vilib>:"Application Directory.vi"() -> ("Application Directory"=w1289:path)
            n282 = Format Date/Time String(time format string (%c)="%p", seconds (now)=w1293) -> (date/time string=w1291:string)  [unwired: 1 in]
            n283 = Path To String(path=w1289) -> (string=w1286:string)
            n284 = Concatenate Strings(w1286, "\\Alicat Data Log_" ("string"), w1292, "_" ("string"), w1291, ".txt" ("string")) -> (w1287:string)
          }
        }
        n285 = call "Data Logging_Check Validity.vi"("error in"=w1242, "Data Frame Format"=w1248, "Data Logging Options (If valid)"="Data Logging Options") -> ("error out"=w1250:errorcluster, "Invalid data selected"=w1249:bool, "Validated Logging Options"=w1237:T3)  [unwired: 6 in]
        n286 = property on="Data Logging Options" class="Clust (strict)"("Value"=w1237) -> ()  [unwired: 2 in, 2 out]
        n287 = call "Data Logging_Generate Header.vi"("error in"=w1250, "Include Units\nin Header (F)"=TRUE ("Include Units\nin Header (default is F)"), "Units of Measure Input"=w1251, "Data Logging Options"=w1237) -> ("error out"=w1256:errorcluster, "Data Log Header"=w1255:string)  [unwired: 6 in]
        n288 = String To Path(string=w1258) -> (path=w1254:path)
        n289 = case shown="True" w1245 {
          tunnel: [w1275 w1281] -> w1257
          tunnel: w1256 -> [w1275 w1276]
          tunnel: w1255 -> [_ w1280]
          tunnel: w1254 -> [_ w1279]
          tunnel: T21."replace or create" ("operation (0:open)") -> [_ w1278]
          tunnel: [refnum<file> refnum ("refnum out") w1277] -> w1252
          frame False {
          }
          frame True {
            n290 = Open/Create/Replace File(file path (use dialog)=w1279, error in=w1276, operation (0:open)=w1278) -> (refnum out=w1283:refnum<file>, error out=w1282:errorcluster)  [unwired: 3 in, 1 out]
            n291 = Write to Text File(file (use dialog)=w1283, text=w1280, error in=w1282) -> (refnum out=w1277:refnum<file>, error out=w1281:errorcluster)  [unwired: 1 in, 1 out]
          }
        }
        n292 = call "Display Message to User2"("Enable"=w1249) -> ()  [unwired: 9 in, 2 out]
        n293 = Select(t=0, s=w1257, f=w1263) -> (s? t:f=w1264:i32)
      }
    }
    n294 = case shown="True" w70 {
      selector: w70 -> [w99 _]
      tunnel: w73 -> [_ w112]
      tunnel: [w99 FALSE ("Data Changed")] -> w71
      tunnel: w69 -> [w97 w113]
      tunnel: w68 -> [w98 w124]
      tunnel: [w98 w123] -> w67
      tunnel: [w97 w103] -> w51
      tunnel: w65 -> [w96 w120]
      tunnel: [w96 w119] -> w66
      tunnel: w55 -> [_ w114]
      tunnel: w47 -> [_ w102]
      frame False {
      }
      frame True {
        # "Only update if new data is received, only log or plot if enabled"
        n295 = case shown="False" w114 {
          tunnel: w124 -> [w129 w154]
          tunnel: [w129 w153] -> w123
          tunnel: w113 -> [w128 w152]
          tunnel: w112 -> [w127 w147]
          tunnel: [w128 w148] -> w103
          tunnel: [w127 w147] -> w111
          frame False {
          }
          frame True {
            # "If true: generate data\nstring and log it to file"
            n296 = local read "Data Logging Options"() -> (w150:T3)
            n297 = Unbundle(w147) -> ("Absolute Pressure"=w146:dbl, "Gauge/Diff. Pressure"=w145:dbl, "Barometric Pressure"=w144:dbl, "Temperature"=w143:dbl, "Volumetric Flow"=w142:dbl, "Mass Flow"=w141:dbl, "Setpoint"=w140:dbl, "Valve Drive"=w139:dbl, "Totalizer"=w138:dbl, "[h]"=w137:dbl, "[m]"=w136:dbl, "[s]"=w135:dbl, "Totalizer Average Flow"=w131:dbl, "Totalizer Peak Flow"=w132:dbl, "Gas selected"=w133:string)  [unwired: 14 out]
            n298 = Bundle(cluster=T19 {"Absolute Pressure"=0.0, "Gauge/Diff. Pressure"=0.0, "Barometric Pressure"=0.0, "Temperature"=0.0, "Volumetric"=0.0, "Mass Flow"=0.0, "Setpoint"=0.0, "Valve Drive"=0.0, "Totalizer"=0.0, "[hr]"=0.0, "[min]"=0.0, "[sec]"=0.0, "Totalizer Average Flow"=0.0, "Totalizer Peak Flow"=0.0, "Gas selected"=""} ("Measurement Data"), "Absolute Pressure"=w146, "Gauge/Diff. Pressure"=w145, "Barometric Pressure"=w144, "Temperature"=w143, "Volumetric"=w142, "Mass Flow"=w141, "Setpoint"=w140, "Valve Drive"=w139, "Totalizer"=w138, "[hr]"=w137, "[min]"=w136, "[sec]"=w135, "Totalizer Average Flow"=w131, "Totalizer Peak Flow"=w132, "Gas selected"=w133) -> (w130:T19)
            n299 = call "Data Logging_Generate Data String.vi"("error in"=w152, "Measurement Data"=w130, "Data Logging Options"=w150) -> ("error out"=w149:errorcluster, "Data Log String"=w151:string)  [unwired: 6 in, 1 out]
            n300 = Write to Text File(file (use dialog)=w154, text=w151, error in=w149) -> (refnum out=w153:refnum<file>, error out=w148:errorcluster)  [unwired: 1 in, 1 out]
          }
        }
        "Measurement Data" <- w111
        n301 = Unbundle By Name(w102) -> ("Absolute Pressure"=w101:bool)
        n302 = Unbundle By Name(w111) -> ("Absolute Pressure"=w109:dbl, "Gauge/Diff. Pressure"=w100:dbl, "Temperature"=w107:dbl, "Volumetric Flow"=w106:dbl, "Mass Flow"=w105:dbl, "Setpoint"=w104:dbl)
        n303 = call "Elapsed Time"("Set Start Time (s)"=w120) -> ("Get Start Time (s)"=w119:dbl, "Elapsed Time (s)"=w116:dbl)  [unwired: 11 in, 6 out]
        n304 = Select(t=w109, s=w101, f=w100) -> (s? t:f=w108:dbl)
        n305 = Multiply(x=1000.0, y=w116) -> (x*y=→"Time between\nreadings [ms]":dbl)
        n306 = Reciprocal(x=w116) -> (1/x=→"Meas. per\nsecond [Hz]":dbl)
        n307 = Bundle(cluster=T5 {"Pressure"=0.0, "Temperature"=0.0, "Volumetric"=0.0, "Mass"=0.0, "SetPoint"=0.0} ("Chart"), "Pressure"=w108, "Temperature"=w107, "Volumetric"=w106, "Mass"=w105, "SetPoint"=w104) -> (w122:T5)
        n308 = case shown="True" "Chart: Graphing" {
          tunnel: w122 -> [_ w126]
          frame False {
          }
          frame True {
            "Chart" <- w126
          }
        }
      }
    }
    n309 = Select(t=50, s=w51, f=0) -> (s? t:f=w59:i32)
    n310 = Select(t=w51, s=w51, f=w49) -> (s? t:f=w50:errorcluster)
  }
  n311 = case shown="True" w7 {
    tunnel: w26 -> [_ w1296]
    frame False {
    }
    frame True {
      # "Currently logging"
      n312 = Close File(refnum=w1296) -> ()  [unwired: 1 in, 2 out]
    }
  }
  n313 = Unbundle(w12) -> (w11:refnum<vi>, "Panel"=w10:refnum<vi>)
  n314 = VISA Close(VISA resource name=w45, error in (no error)=w43) -> (error out=w14:errorcluster)
  n315 = Close Reference(reference=w11, error in (no error)=w14) -> (error out=w15:errorcluster)
  n316 = Close Reference(reference=w10, error in (no error)=w15) -> (error out=w13:errorcluster)
  n317 = call <vilib>:"Simple Error Handler.vi"("error in (no error)"=w13) -> ()  [unwired: 4 in, 5 out]
